vi "myRIOSpecPage_Template.vi"(10 "Spec Page Interface":T2, 11 "MetaDataObj in":refnum<class "MetaDataObj.lvclass">) -> (3 "MetaDataObj out":refnum<class "MetaDataObj.lvclass">)   [LabVIEW 2021, in "myRIOMetaDataObj.lvclass"]
uses:
  myRIOMetaDataObj.lvclass
  <resource>/dialog/NewProjectWizard/Icon Overlay/NI_NPW_Icon Overlay.lvlib
  <resource>/myRIO/Target Info.ctl
  WizardUIRef.ctl
  TargetListInfo.ctl
  TargetInfoHistory.ctl
  <vilib>/Utility/miscctls.llb/LVSelectionTypeDef.ctl
  AvailableTargets.ctl
  InternalErrorCodes.vi
  ModeFunctionality.ctl
  <vilib>/myRIO/Common/Instrument Driver Framework/Utilities/xctls/myRIO Device Button/myRIO Device Button.xctl
  <resource>/dialog/NewProjectWizard/MetaDataObj/MetaDataObj.lvclass
  <vilib>/Utility/cursorutil.llb/Set Cursor (Icon Pict).vi
  <vilib>/Platform/browser.llb/Open URL in Default Browser (string).vi
  p:/lvdist/win32/export/21.0/21.0.0f0/dist/resource/dialog/NewProjectWizard/MetaDataObj/MetaDataObj.lvclass
  p:/lvdist/win32/export/21.0/21.0.0f0/dist/ProjectTemplates/Source/myRIO/scripting/myRIOMetaDataObj/myRIOMetaDataObj.lvclass
  <resource>/dialog/NewProjectWizard/Spec Page Interface Confirm Quit.ctl
panel:
  in  "Project Name":string
  in  "Project Root":path
  in  "File Name Prefix (Optional)":string
  out "FPGA Personality Indicator":string
  out "myRIO Device Button":bool(xcontrol)
  in  "Personality Tags":u16(ring) items=["myRIO_FP_Default", "myRIO_FP_Throughput"]
  out "Mode Help Link":string
  out "FunctionalityArray":T1[](array[typedef])
  in  "FPGA Personality Selector":u16(ring) items=["Default", "High Throughput"]
  in  "Refresh Button":bool
  in  "Target Tab Control":enum32{"Target List Page", "IP Config Page"}(tab)
  in  "TargetList":i32(listbox) caption="Target List"
  in  "IP":string caption="IP Address or Hostname :"
  out "WarningMsg":string
  in  "AvailableTargets":T3
  # "Target"
  # "FPGA Personality"
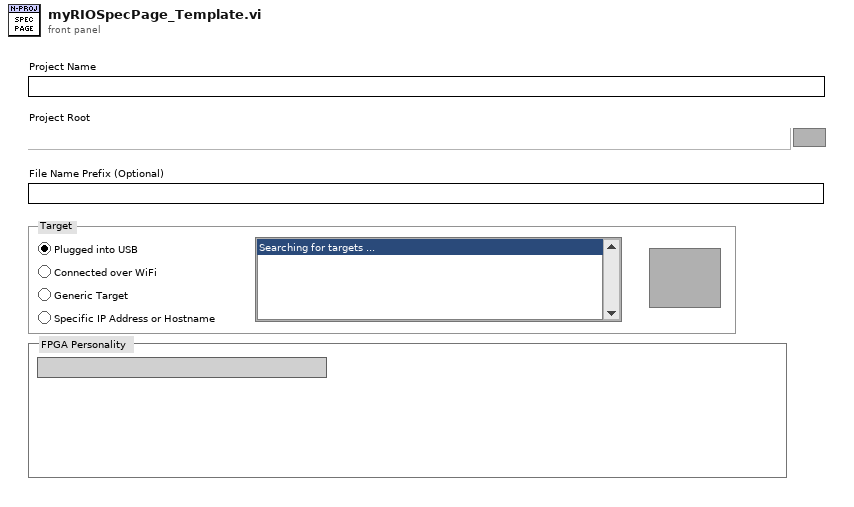
[diagram p1: front panel]
types:
  T1 = typedef "myRIOMetaDataObj.lvclass/ModeFunctionality.ctl" = cluster{"myRIOMode Functionality":u16, "SupportNumber":string}
  T2 = typedef "Spec Page Interface Confirm Quit.ctl" = cluster{"\"Tab Forward To\" Refnum":refnum<vi>, "\"Tab Backward To\" Refnum":refnum<vi>, "Errors":refnum<user-event>, "Quit":refnum<user-event>, "Additional Data":variant}
  T3 = typedef "myRIOMetaDataObj.lvclass/AvailableTargets.ctl" = enum32{"USBTarget", "WifiTarget", "NoSpecificTarget", "TargetIP"}
  T4 = typedef "myRIOMetaDataObj.lvclass/TargetInfoHistory.ctl" = cluster{"USBTargetList":T5, "WiFiTargetList":T5, "GenericTargetList":T5, "IPTargetList":cluster{"IP Error Out":errorcluster, "Target RT Info List":T6[]}}
  T5 = typedef "myRIOMetaDataObj.lvclass/TargetListInfo.ctl" = cluster{"TargetList":string[], "Value":i32, "Target RT Info List":T6[]}
  T6 = typedef "Target Info.ctl" = cluster{"MACAddr":string, "Hostname":string, "IPAddr":string, "SerialNum":string, "ProdID":u32}
  T7 = typedef "myRIOMetaDataObj.lvclass/WizardUIRef.ctl" = cluster{"Project Name":refnum<vi>, "Project Root":refnum<vi>, "File Name Prefix (Optional)":refnum<vi>, "AvailableTargets":refnum<vi>, "Target Tab Control":refnum<vi>, "TargetList":refnum<vi>, "IP":refnum<vi>, "Refresh":refnum<vi>, "FPGA Personality Selector":refnum<vi>, "FPGA Personality Indicator":refnum<vi>}
  T8 = cluster{"Quit":refnum<user-event>, "InitUI":refnum<user-event>, "ValidateUI":refnum<user-event>, "Show Overlay":refnum<user-event>, "Update Path":refnum<user-event>, "UpdateUI":refnum<user-event>}
  T9 = typedef "LVSelectionTypeDef.ctl" = cluster{"Selection Start":u32, "Selection End":u32}
  T10 = enum16{"Initial", "Get Channel Info Index by Name", "Get Channel Info by Index", "Get Channel Info by Img Index"}
  T11 = enum8{"Enabled", "Disabled", "Disabled and Grayed Out"}
  T12 = enum32{"USBTarget", "WifiTarget", "NoSpecificTarget", "TargetIP"}
  T13 = typedef "myRIOMetaDataObj.lvclass/IODetail.ctl" = cluster{"Channel Info Index":i8, "IO Number":i8}
  T14 = typedef "myRIOMetaDataObj.lvclass/ChannelInfo.ctl" = cluster{"Priority":u16, "Channel Shortcut":string, "Channel Description":string, "Channl Image Index":u16}
  T15 = typedef "LVPoint32TypeDef.ctl" = cluster{"Horizontal":i32, "Vertical":i32}
  T16 = typedef "lveventtype.ctl" = enum32{"Null", "Timeout", "Annotation Menu Selection", "Annotation Menu Selection?", "App Instance Close", "App Instance Close?", "Autoscale Range Change", "Bookmark Info Change", "Cell Edit", "Cell Edit?", "Cursor Grab", "Cursor Grab?", "Cursor Menu Selection", "Cursor Menu Selection?", "Cursor Move", "Cursor Release", "Data Change", "Direction Change", "Display State Change", "Drag Ended", "Drag Enter", "Drag Leave", "Drag Over", "Drag Source Update", "Drag Starting", "Drag Starting?", "Drop", "Exec State Change", "Key Down", "Key Down?", "Key Repeat", "Key Repeat?", "Key Up", "Listbox Double Click", "Menu Activation?", "Menu Selection (App)", "Menu Selection? (App)", "Menu Selection (User)", "Mouse Down", "Mouse Down?", "Mouse Enter", "Mouse Leave", "Mouse Move", "Mouse Up", "Mouse Wheel", "NI Security User Change (App)", "Pane Size", "Panel Close", "Panel Close?", "Panel Resize", "Plot Attribute Change", "Scale Range Change", "Shortcut Menu Activation?", "Shortcut Menu Selection (App)", "Shortcut Menu Selection? (App)", "Shortcut Menu Selection (User)", "Tree Double Click", "Tree Drag", "Tree Drag?", "Tree Drop", "Tree Drop?", "Tree Item Close", "Tree Item Close?", "Tree Item Open", "Tree Item Open?", "User Event", "Value Change"}
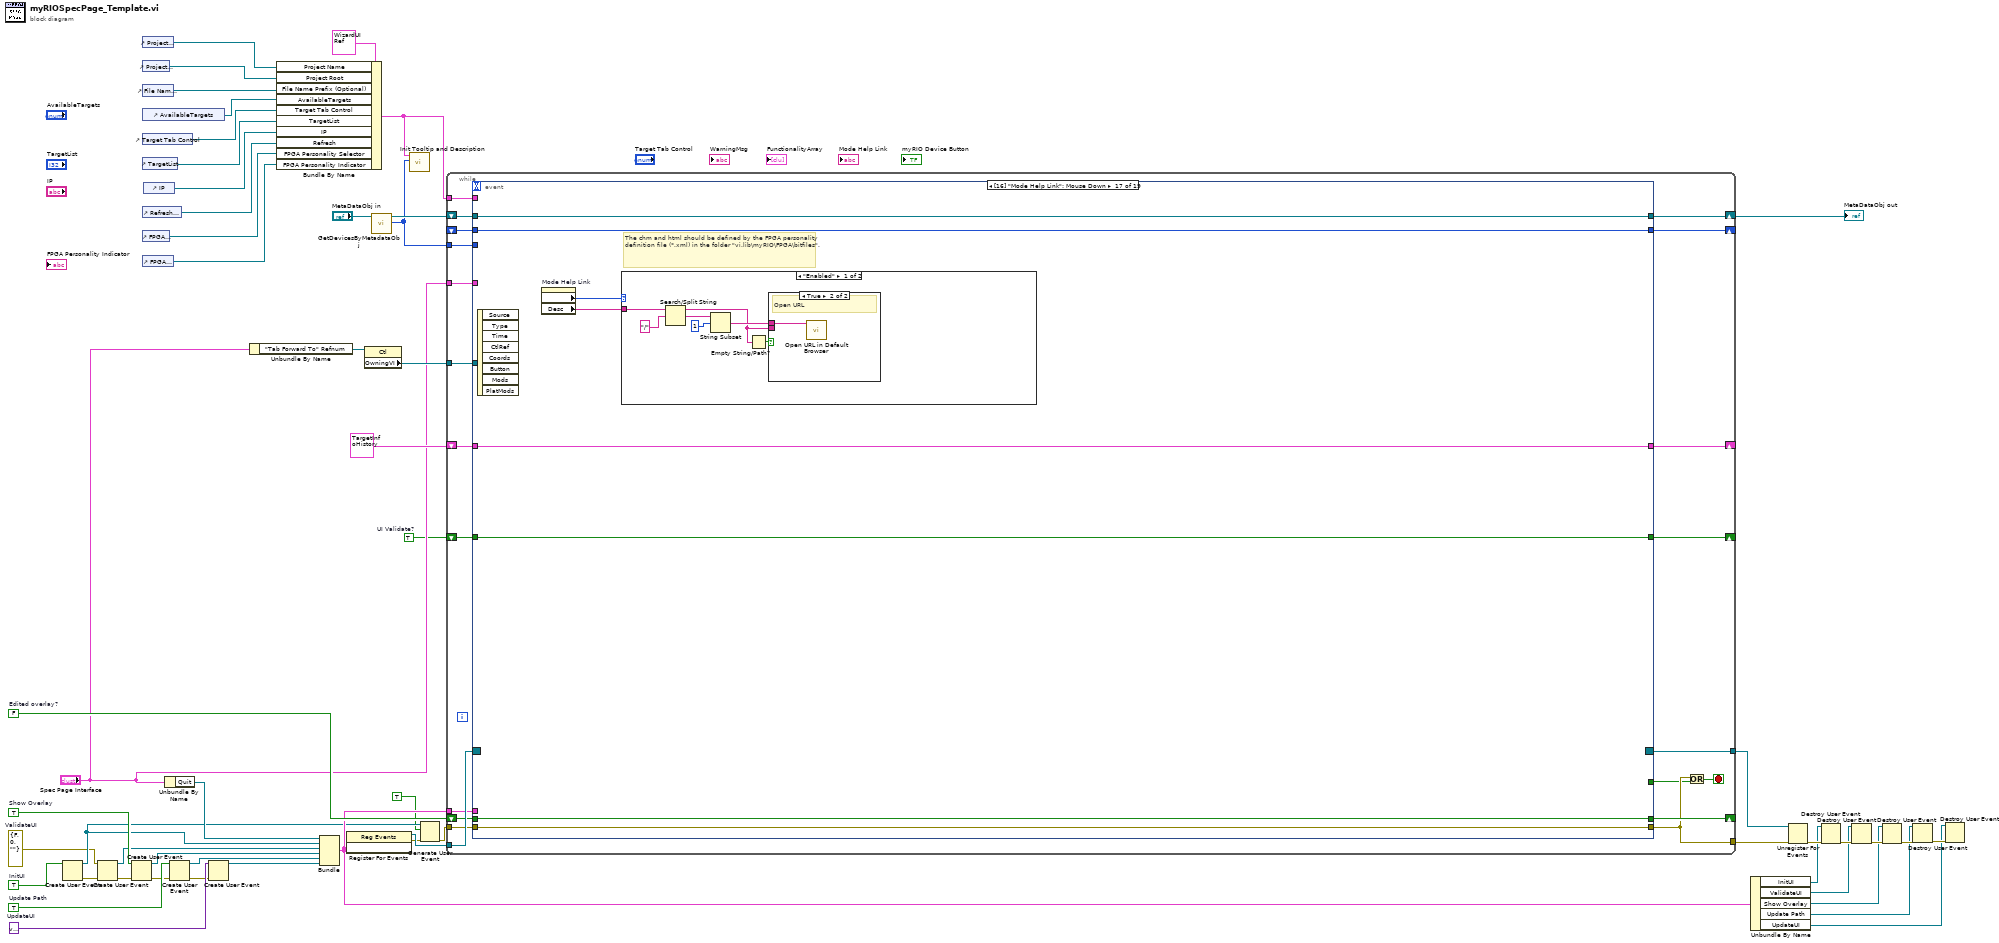
[diagram p0: block diagram]
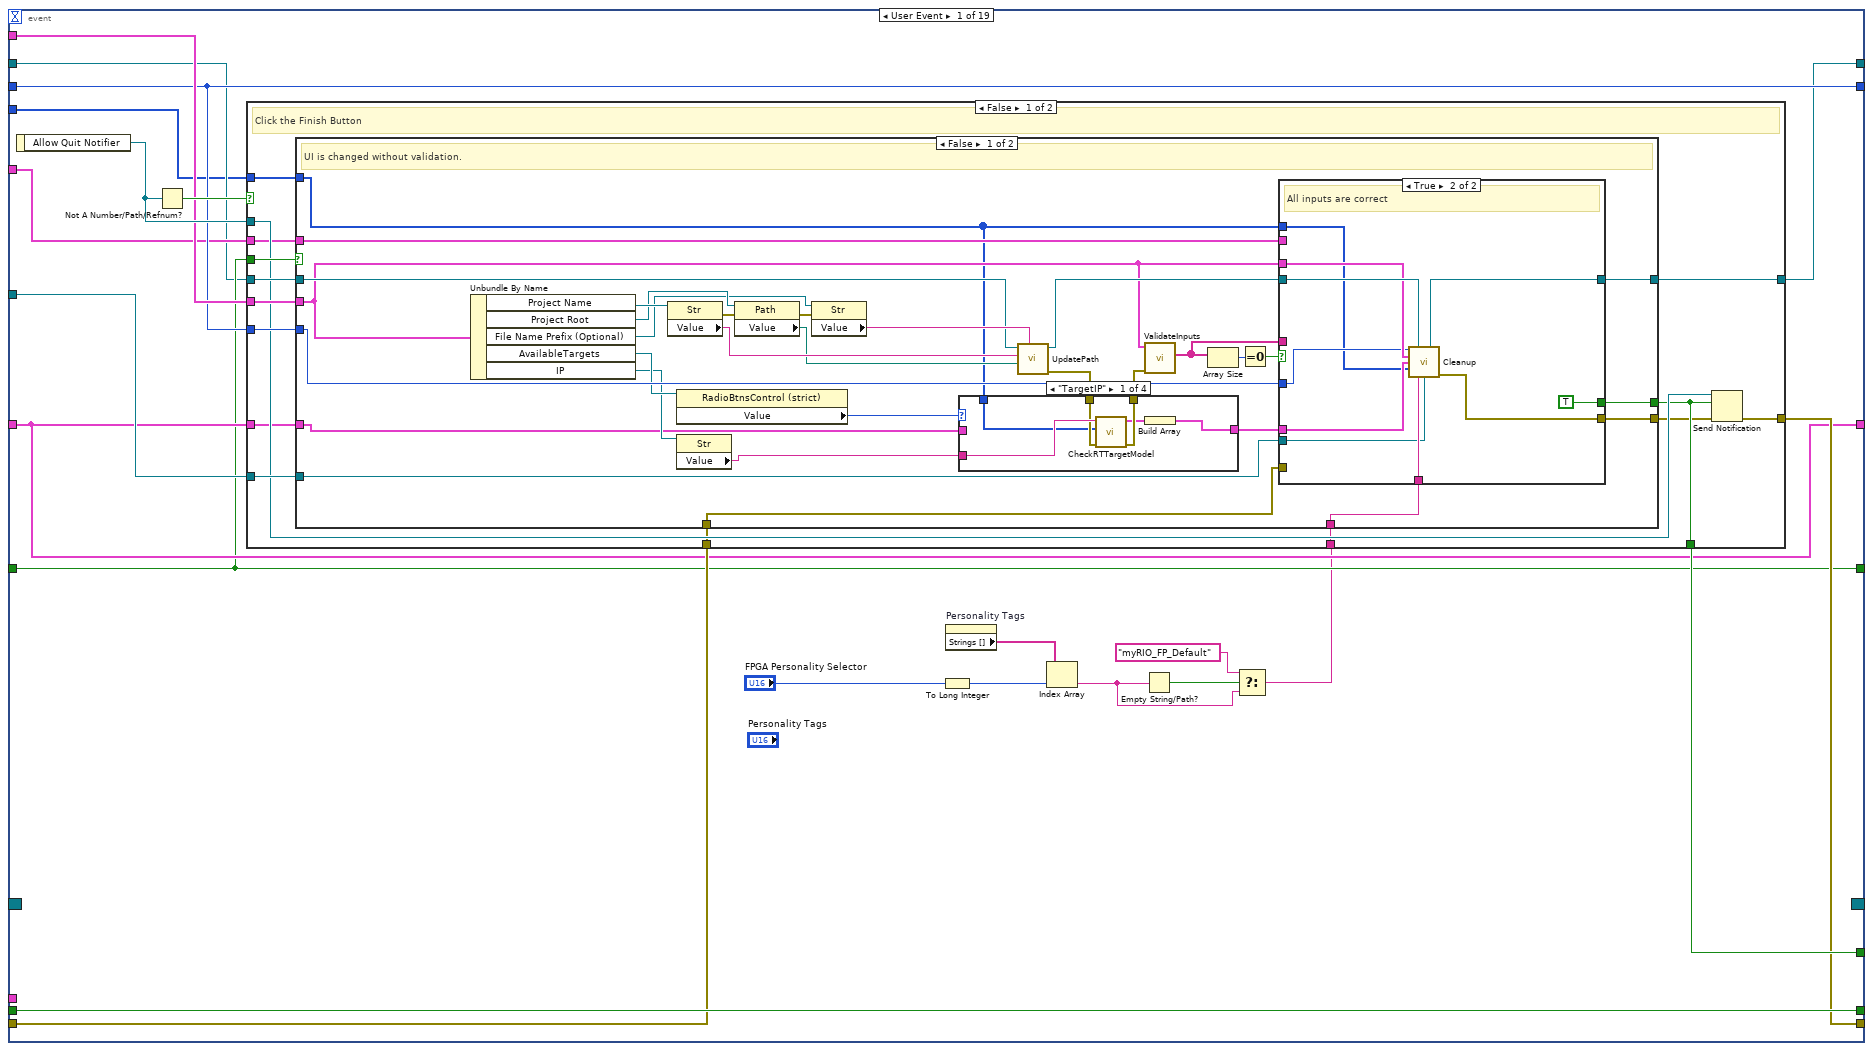
[diagram p2: hidden frame]
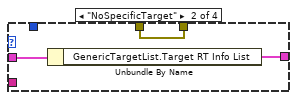
[diagram p3: hidden frame]
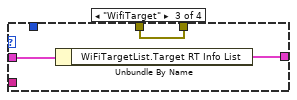
[diagram p4: hidden frame]
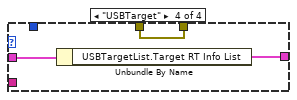
[diagram p5: hidden frame]
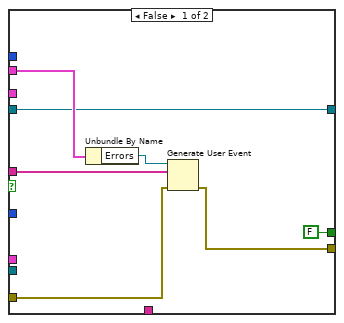
[diagram p6: hidden frame]
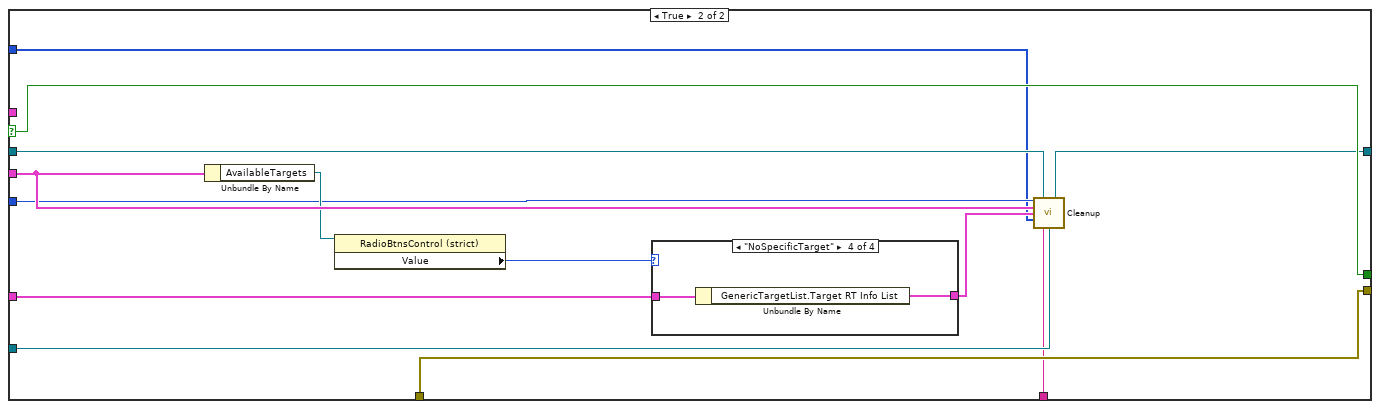
[diagram p7: hidden frame]
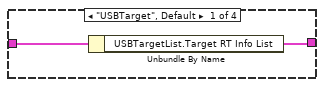
[diagram p8: hidden frame]
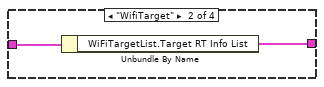
[diagram p9: hidden frame]
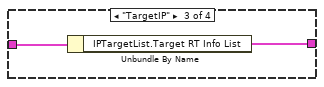
[diagram p10: hidden frame]
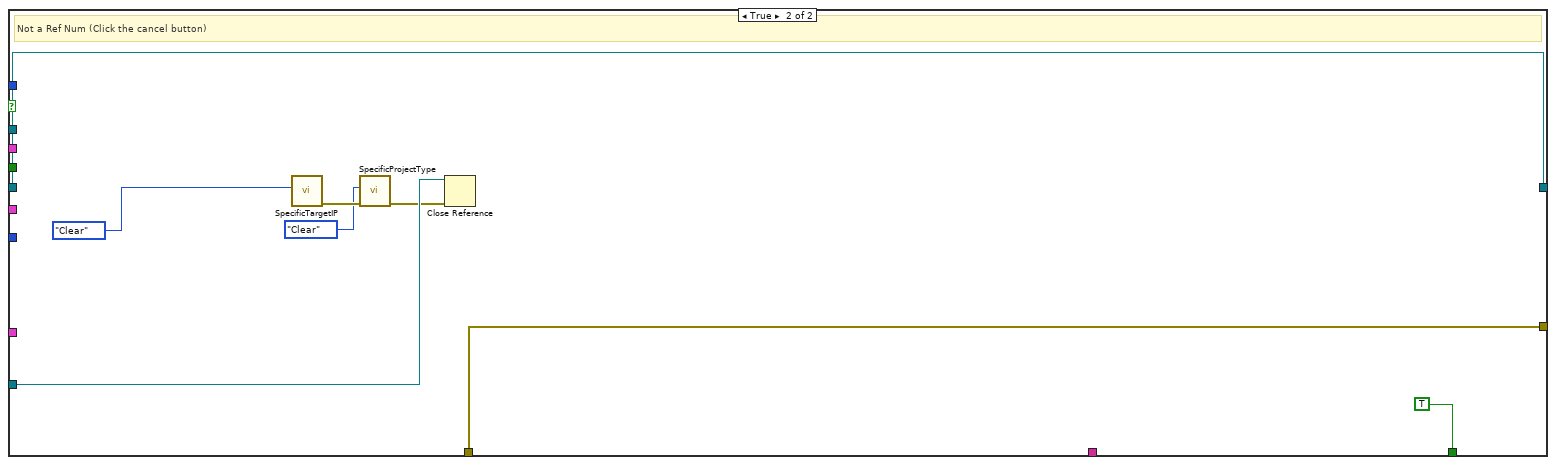
[diagram p11: hidden frame]
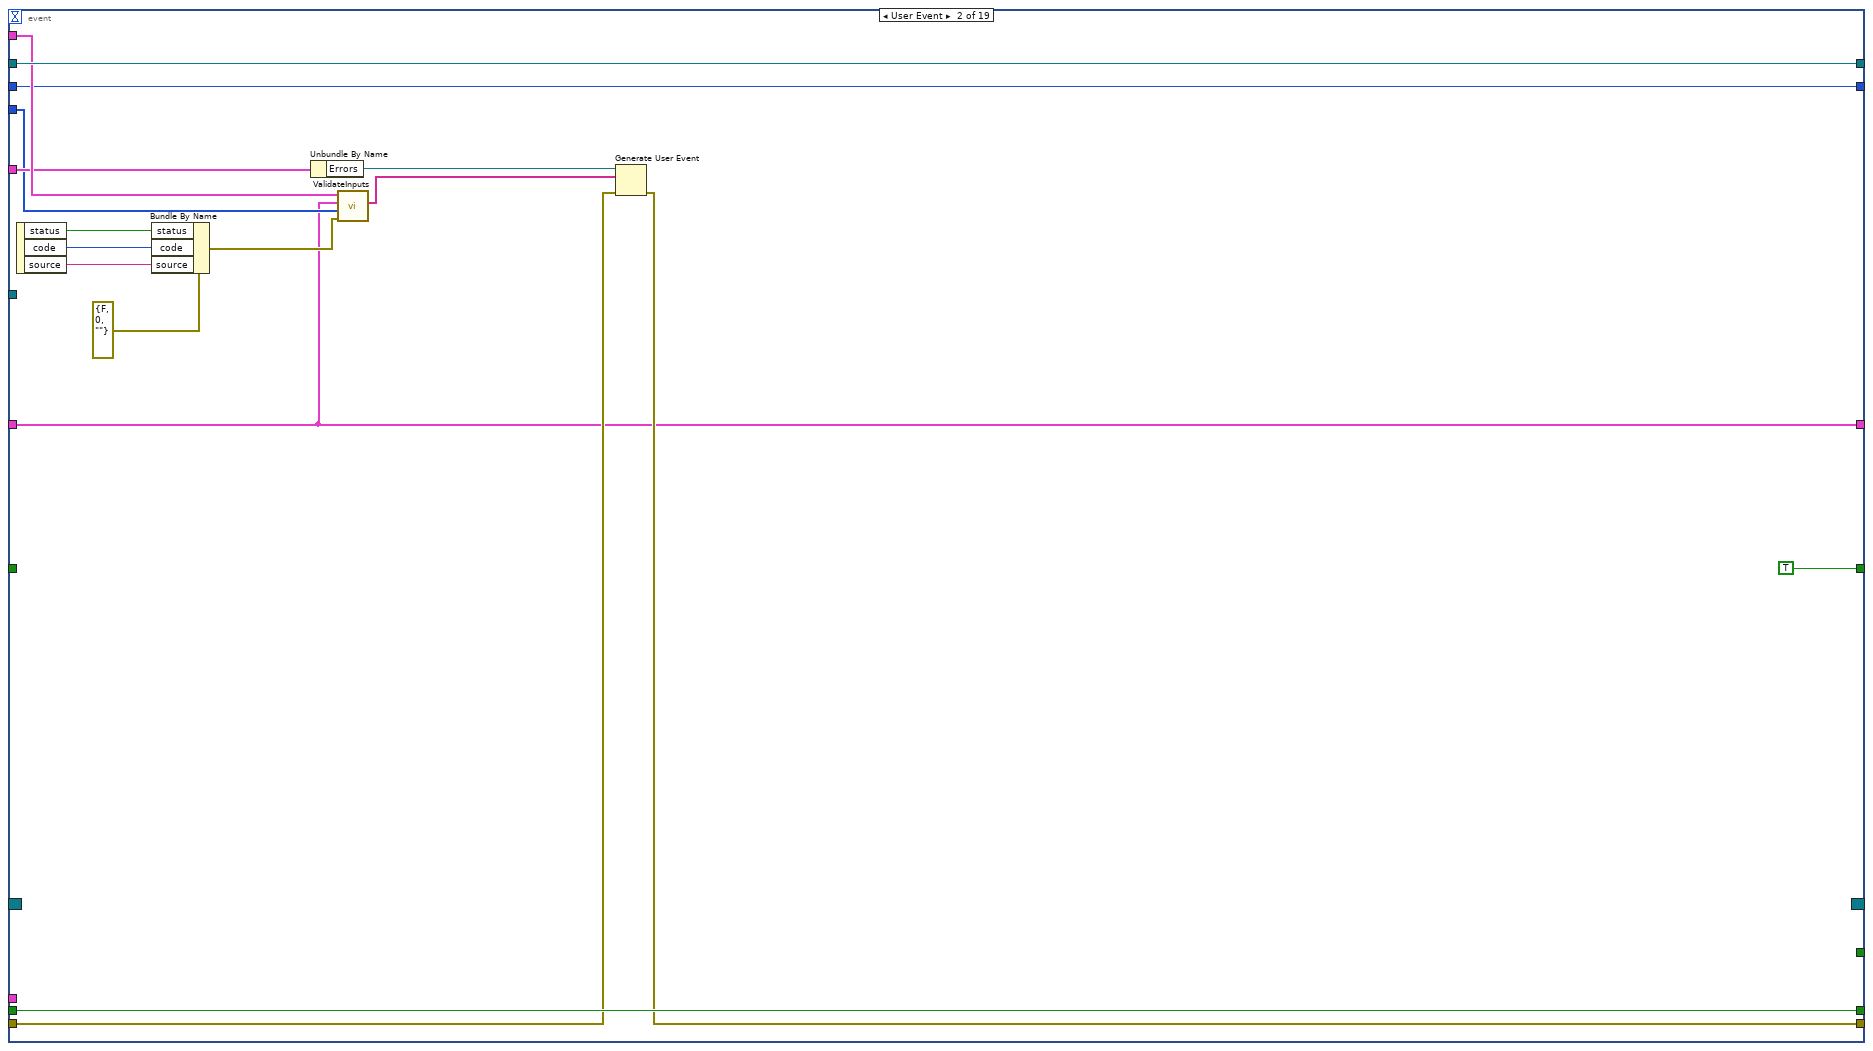
[diagram p12: hidden frame]
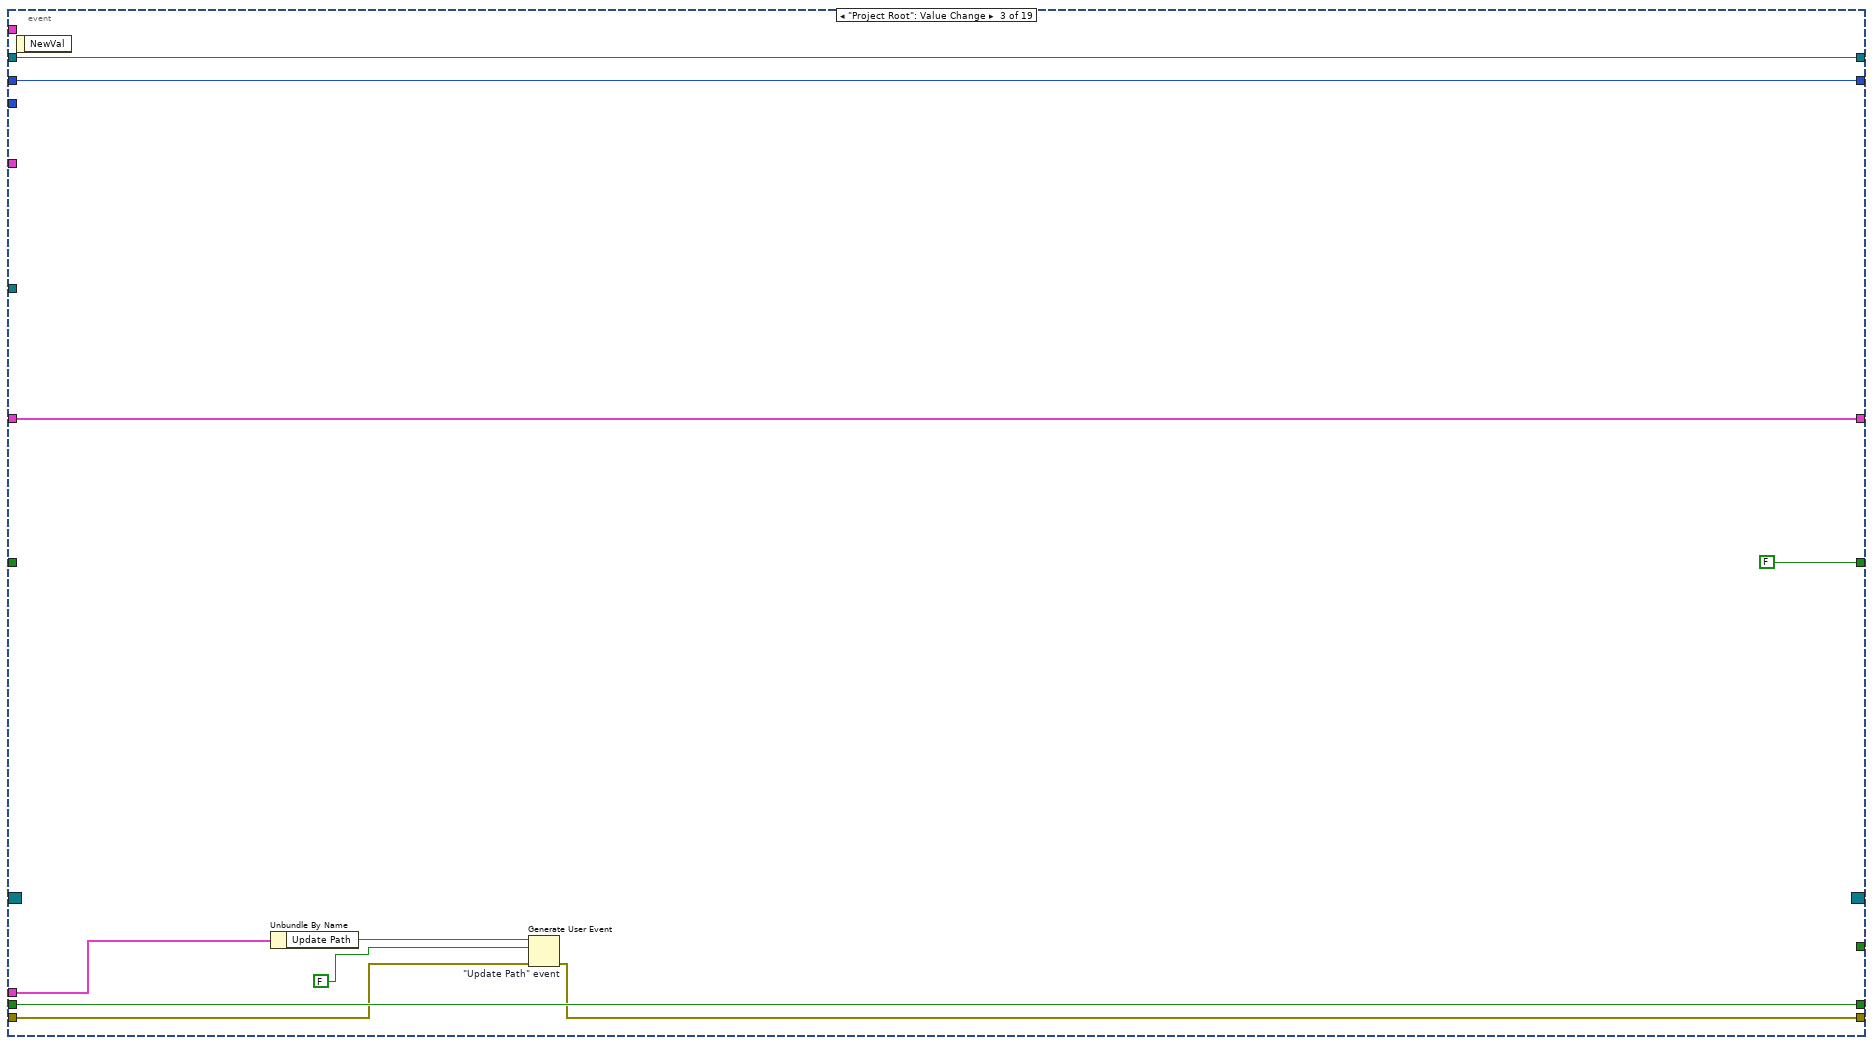
[diagram p13: hidden frame]
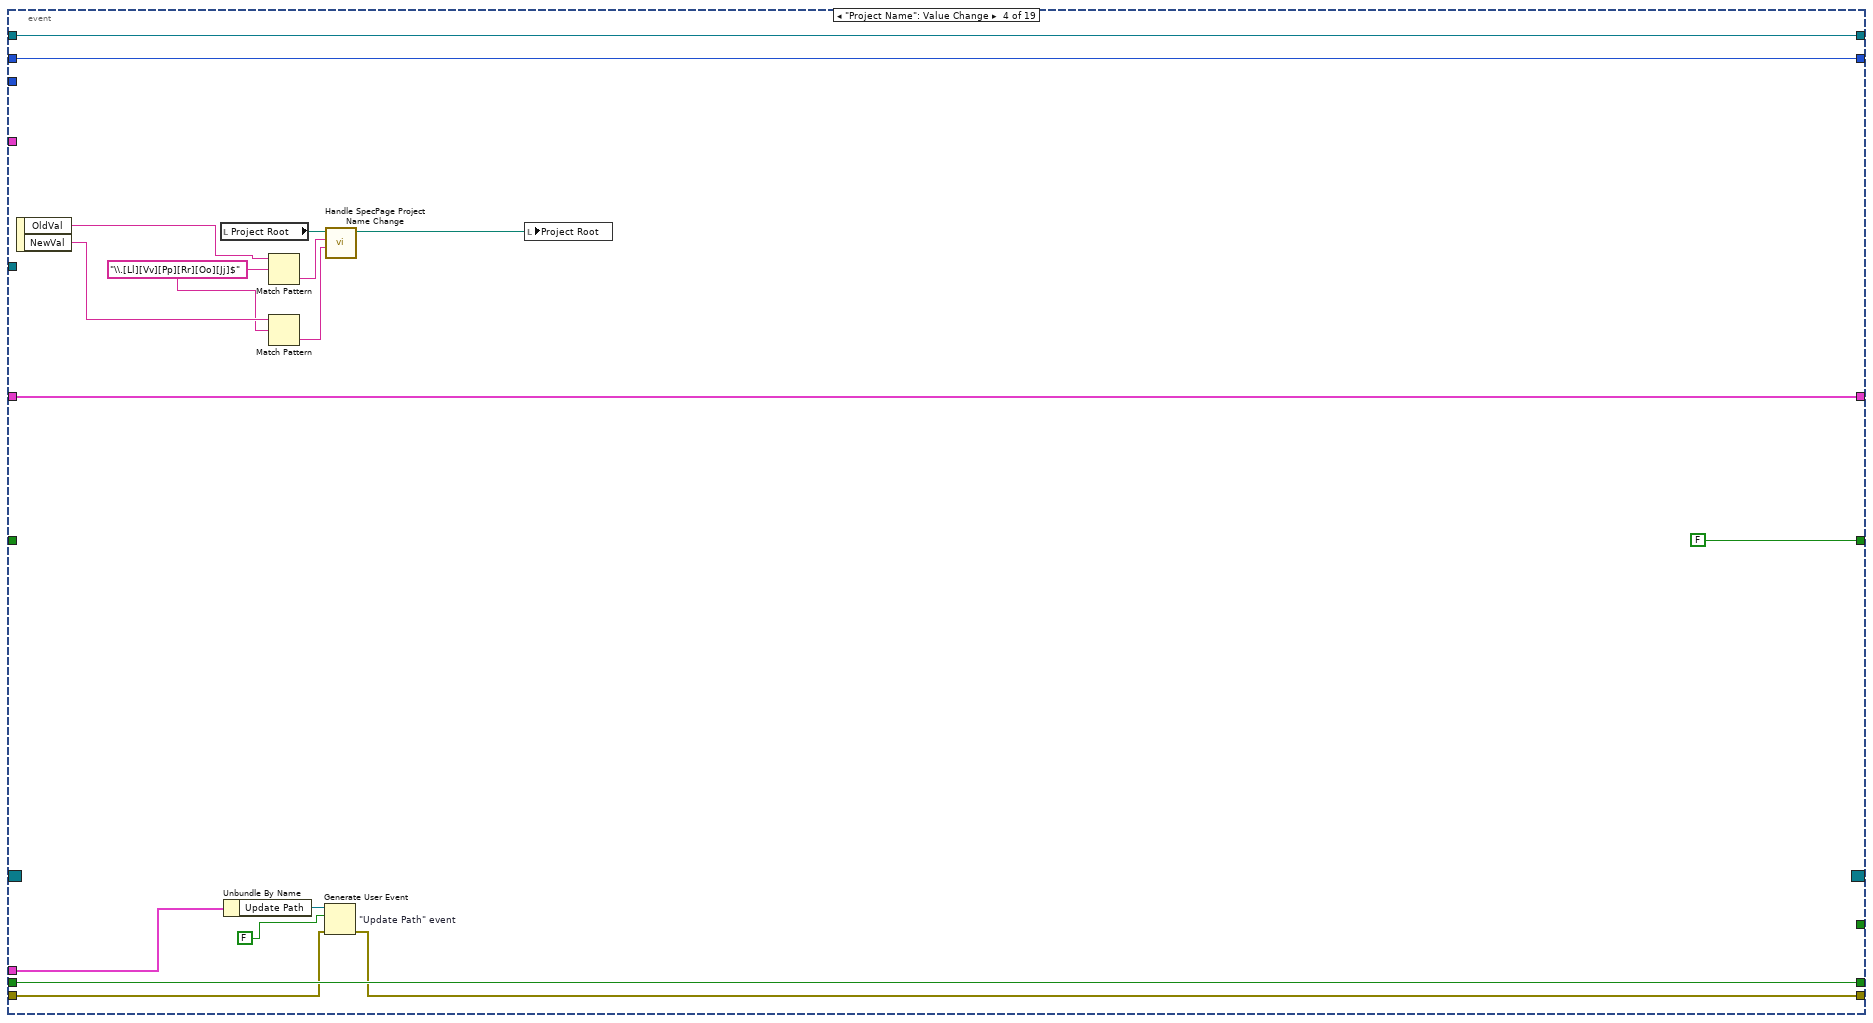
[diagram p14: hidden frame]
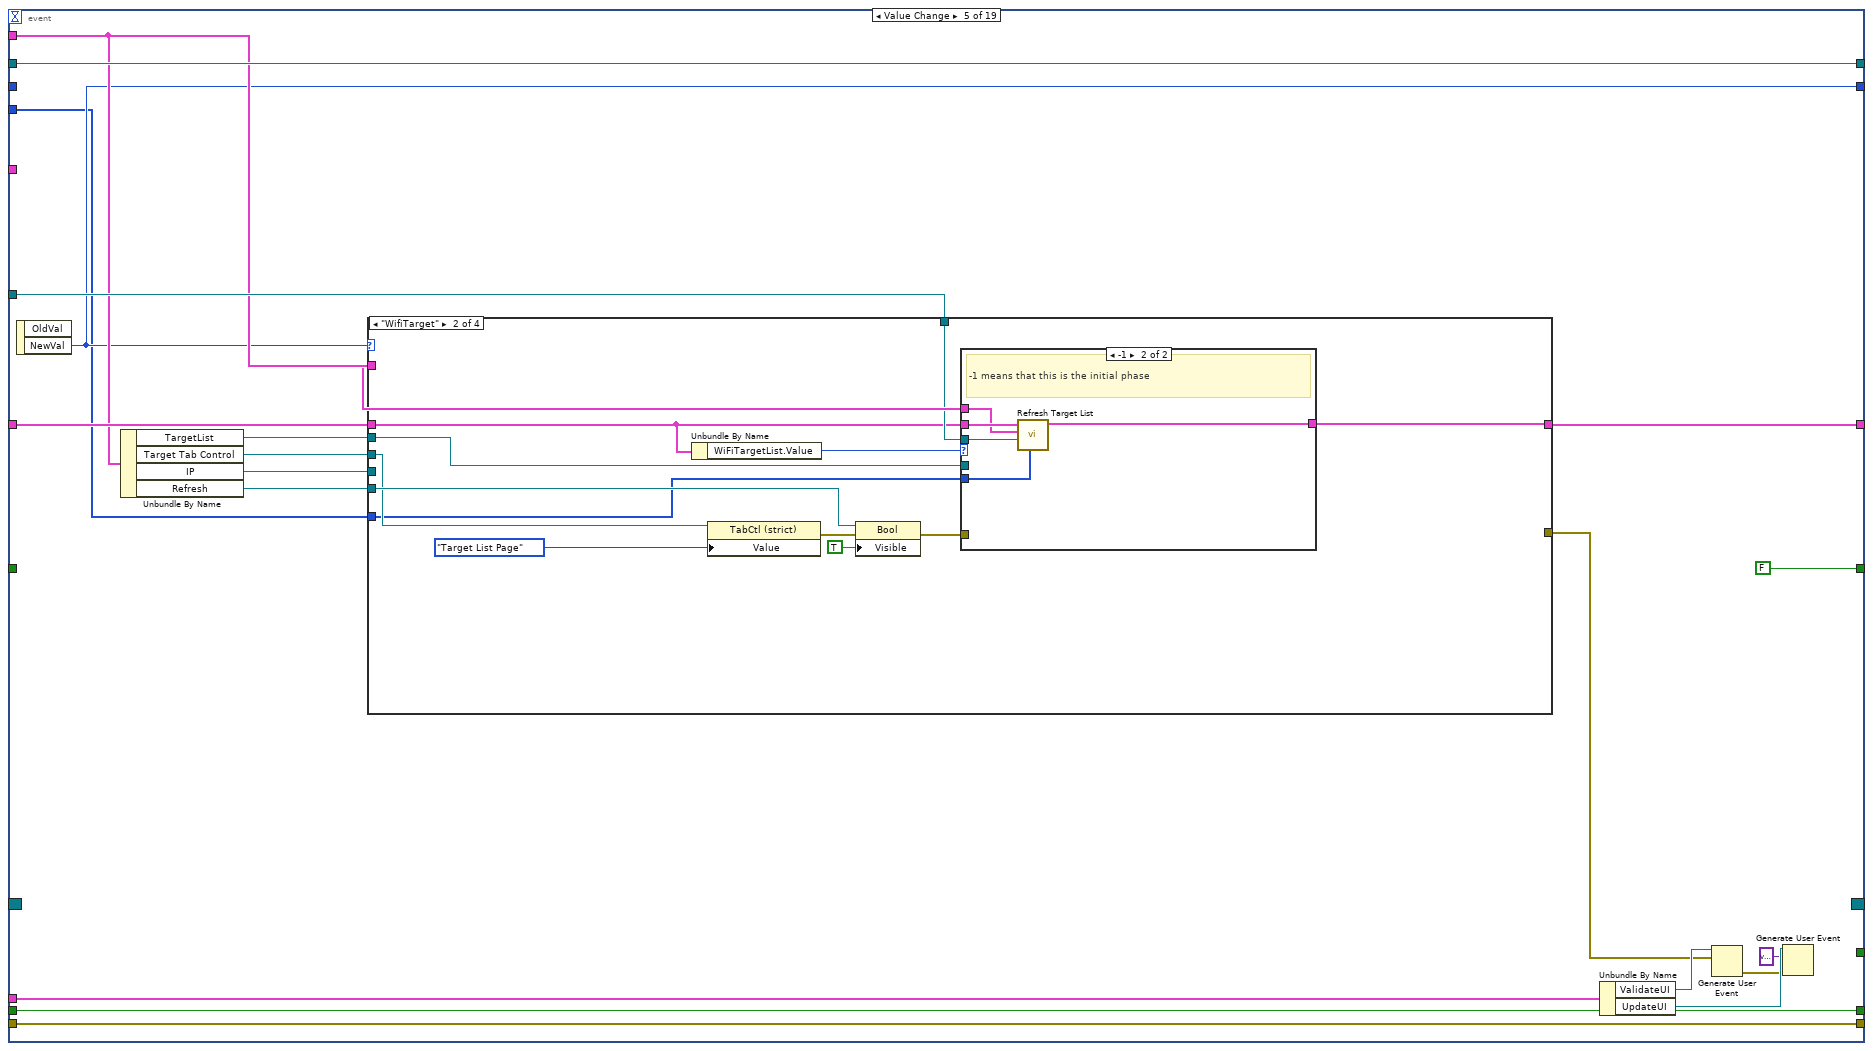
[diagram p15: hidden frame]
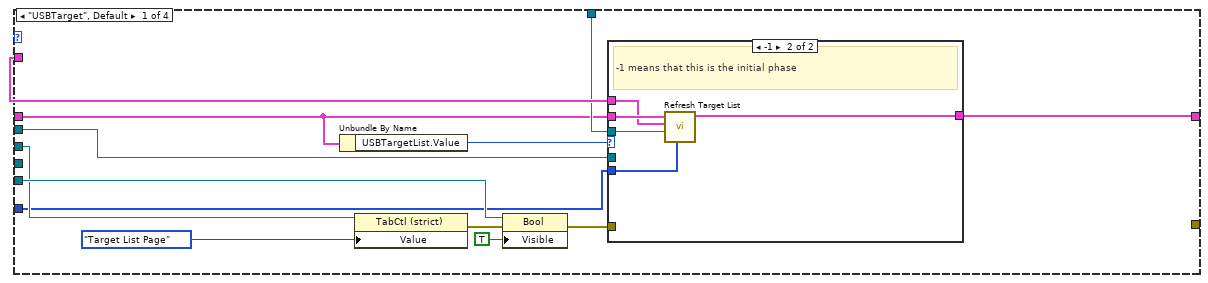
[diagram p16: hidden frame]
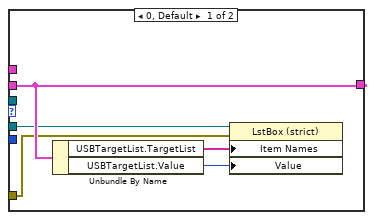
[diagram p17: hidden frame]
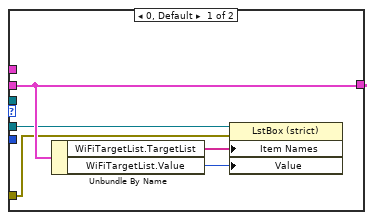
[diagram p18: hidden frame]
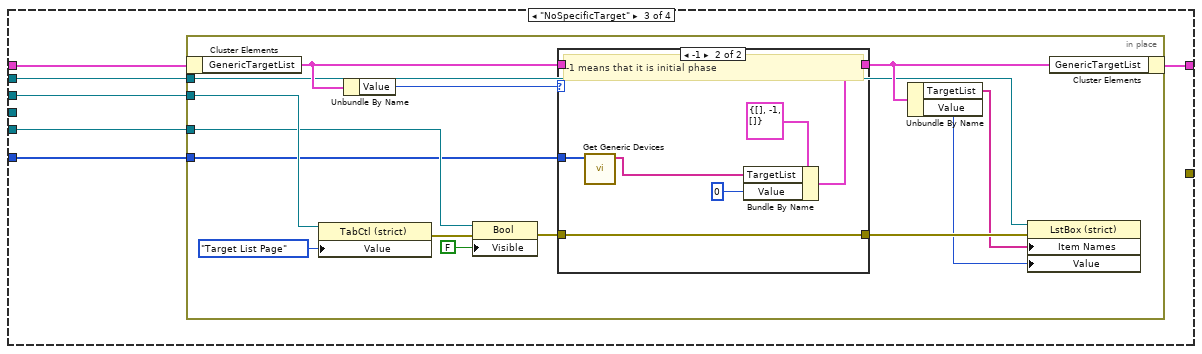
[diagram p19: hidden frame]
diagram:
  w12 = variant  # UpdateUI
  w15 = TRUE  # UI Validate?
  w14 = errorcluster {"status"=FALSE, "code"=0, "source"=""}  # ValidateUI
  w46 = TRUE  # InitUI
  w49 = FALSE  # Edited overlay?
  w48 = TRUE  # Show Overlay
  w53 = TRUE  # Update Path
  n1 = Create User Event(user event datatype=w46) -> (user event=w22:refnum<user-event>, error out=w45:errorcluster)  [unwired: 1 in]
  n2 = Create User Event(user event datatype=w14, error in=w45) -> (user event=w42:refnum<user-event>, error out=w44:errorcluster)
  n3 = Create User Event(user event datatype=w48, error in=w44) -> (user event=w41:refnum<user-event>, error out=w43:errorcluster)
  n4 = control-ref of="Project Name"() -> (w33:refnum<vi>)
  n5 = control-ref of="Project Root"() -> (w34:refnum<vi>)
  n6 = control-ref of="File Name Prefix (Optional)"() -> (w35:refnum<vi>)
  n7 = control-ref of="AvailableTargets"() -> (w7:refnum<vi>)
  n8 = control-ref of="Target Tab Control"() -> (w36:refnum<vi>)
  n9 = control-ref of="TargetList"() -> (w37:refnum<vi>)
  n10 = control-ref of="Refresh Button"() -> (w13:refnum<vi>)
  n11 = control-ref of="FPGA Personality Selector"() -> (w6:refnum<vi>)
  n12 = control-ref of="FPGA Personality Indicator"() -> (w5:refnum<vi>)
  n13 = control-ref of="IP"() -> (w38:refnum<vi>)
  n14 = Unbundle By Name("Spec Page Interface") -> ("Quit"=w39:refnum<user-event>)
  n15 = Create User Event(user event datatype=w53, error in=w43) -> (user event=w40:refnum<user-event>, error out=w11:errorcluster)
  n16 = Create User Event(user event datatype=w12, error in=w11) -> (user event=w10:refnum<user-event>)  [unwired: 1 out]
  n17 = Unbundle By Name("Spec Page Interface") -> ("\"Tab Forward To\" Refnum"=w20:refnum<vi>)
  n18 = Bundle By Name(cluster=T7 {"Project Name"=refnum, "Project Root"=refnum, "File Name Prefix (Optional)"=refnum, "AvailableTargets"=refnum, "Target Tab Control"=refnum, "TargetList"=refnum, "IP"=refnum, "Refresh"=refnum, "FPGA Personality Selector"=refnum, "FPGA Personality Indicator"=refnum} ("output cluster"), "Project Name"=w33, "Project Root"=w34, "File Name Prefix (Optional)"=w35, "AvailableTargets"=w7, "Target Tab Control"=w36, "TargetList"=w37, "IP"=w38, "Refresh"=w13, "FPGA Personality Selector"=w6, "FPGA Personality Indicator"=w5) -> (w4:T7)
  n19 = Bundle("Quit"=w39, "InitUI"=w22, "ValidateUI"=w42, "Show Overlay"=w41, "Update Path"=w40, "UpdateUI"=w10) -> (w31:T8)  [unwired: 1 in]
  n20 = register-events(w31) -> (reference out=w54:refnum<event-registration>, error out=w24:errorcluster)  [unwired: 2 in]
  n21 = property class="Ctl"(reference=w20) -> ("OwningVI"=w19:refnum<vi>)  [unwired: 1 in, 2 out]
  n22 = call "GetDevicesByMetadataObj.vi"("MetaDataObj in"="MetaDataObj in") -> ("Supported Devices"=w3:u32[], "MetaDataObj Out"=w8:refnum<class "MetaDataObj.lvclass">)  [unwired: 7 in, 2 out]
  n23 = call "Init Tooltip and Description.vi"("Supported Devices"=w3, "Main UI Ref Cluster"=w4) -> ()  [unwired: 10 in]
  n24 = Generate User Event(user event=w22, event data cluster=TRUE ("event data"), error in=w24) -> (error out=w23:errorcluster)  [unwired: 1 in, 1 out]
  n25 = while {
    tunnel: "Spec Page Interface" -> [w74]
    shift-right: [w73] -> w51
    shift-left: w8 -> [w72]
    tunnel: w54 -> [w75]
    shift-right: [w69] -> _
    shift-left: w49 -> [w70]
    shift-right: [w68] -> _
    shift-left: _ -> [w67]
    tunnel: w23 -> [w66]
    tunnel: w4 -> [w63]
    tunnel: [w65] -> w47
    tunnel: w31 -> [w64]
    tunnel: w19 -> [w62]
    tunnel: [w61] -> w18
    shift-right: [w59] -> _
    shift-left: T4 {"USBTargetList"={"TargetList"=[], "Value"=-1, "Target RT Info List"=[]}, "WiFiTargetList"={"TargetList"=[], "Value"=-1, "Target RT Info List"=[]}, "GenericTargetList"={"TargetList"=[], "Value"=-1, "Target RT Info List"=[]}, "IPTargetList"={"IP Error Out"={"status"=FALSE, "code"=0, "source"=""}, "Target RT Info List"=[]}} ("TargetInfoHistory") -> [w60]
    shift-right: [w58] -> _
    shift-left: w15 -> [w57]
    tunnel: w3 -> [w55]
    stop <- w71 stop-if-true
    n26 = event shown="[16] \"Mode Help Link\": Mouse Down" {
      selector: w75 -> [_ _ _ _ _ _ _ _ _ _ _ _ _ _ _ _ _ _ _]
      dyn-events: [_ _ _ _ _ _ _ _ _ _ _ _ _ _ _ _ _ _ _] -> w61
      timeout: _ -> [_ _ _ _ _ _ _ _ _ _ _ _ _ _ _ _ _ _ _]
      tunnel: w74 -> [w86 w216 _ _ _ _ _ _ _ _ w634 _ _ _ _ _ _ _ _]
      tunnel: [w89 w215 w224 w235 w266 w397 w485 w520 w582 w609 w635 w659 w664 w693 w762 w805 w813 w837 w875] -> w65
      tunnel: [w91 w221 w231 w244 w267 w383 w502 w536 w591 w602 w638 w662 w668 w695 w757 w804 w812 w836 w874] -> w73
      tunnel: w72 -> [w81 w221 w231 w244 w267 w410 w502 w536 w592 w603 w638 w662 w668 w695 w757 w804 w812 w836 w874]
      tunnel: w70 -> [w97 w220 w229 w245 w268 w427 w501 w537 w590 w614 w637 w661 w667 w694 w761 w803 w811 w835 w873]
      tunnel: [w97 w220 w229 w245 w268 w427 w501 w537 w590 w614 w637 w661 w667 w694 w761 w803 w811 w835 w873] -> w69
      tunnel: [w93 w214 w228 w238 w254 w396 w488 w526 w589 w613 w636 w650 w663 w687 w758 w802 w810 w834 w872] -> w68
      tunnel: w67 -> [w93 w214 w228 w238 _ _ w488 w526 w589 w613 w636 w650 w663 w687 w758 w802 w810 w834 w872]
      tunnel: w66 -> [w88 w213 w225 w234 w266 w380 w498 w533 w583 w610 w635 w660 w664 w693 w762 w805 w813 w837 w875]
      tunnel: w64 -> [_ _ w227 w237 w264 w405 w500 w535 w588 w612 _ w658 _ _ _ _ _ _ _]
      tunnel: w63 -> [w94 w217 _ _ w261 w393 w497 _ _ _ w633 w655 _ _ _ _ _ _ _]
      tunnel: w62 -> [w92 _ _ _ w265 w400 _ w532 _ _ _ w654 _ _ _ _ _ _ w868]
      tunnel: w60 -> [w87 w205 w223 w233 w263 w398 w493 w530 w581 w607 w632 w652 w666 w686 w759 w801 w808 w833 w871]
      tunnel: [w87 w205 w223 w233 w255 w398 w490 w527 w581 w607 w632 w651 w666 w686 w759 w801 w808 w833 w871] -> w59
      tunnel: [w82 TRUE FALSE ("UI Validate?") FALSE ("UI Validate?") FALSE FALSE ("UI Validate?") w494 FALSE ("UI Validate?") FALSE ("UI Validate?") w608 w631 FALSE ("UI Validate?") FALSE ("UI Validate?") w692 w760 w800 w809 w832 w870] -> w58
      tunnel: w57 -> [w82 _ _ _ _ _ _ _ _ w608 w631 _ _ w692 w760 w800 w809 w832 w870]
      tunnel: [w90 _ _ _ _ _ _ _ _ _ _ _ _ _ _ _ _ _ _] -> w56
      tunnel: w55 -> [w80 w206 _ _ w249 w377 _ w518 _ _ _ w649 _ w669 w751 _ _ _ _]
      event User Event {
        n27 = event-data() -> ("Allow Quit Notifier"=w95:refnum<notifier>)  [unwired: 1 in]
        n28 = Not A Number/Path/Refnum?(number/path/refnum=w95) -> (NaN/Path/Refnum?=w96:bool)
        n29 = To Long Integer(number="FPGA Personality Selector") -> (32bit integer=w83:i32)
        n30 = property on="Personality Tags" class="Ring (strict)"() -> ("Strings []"=w85:string[])  [unwired: 2 in, 2 out]
        n31 = Index Array(array=w85, index=w83) -> (element=w78:string)
        n32 = Empty String/Path?(string/path=w78) -> (empty?=w79:bool)
        n33 = Select(t="myRIO_FP_Default", s=w79, f=w78) -> (s? t:f=w76:string)
        n34 = case shown="False" w96 {
          tunnel: w82 -> [w112 _]
          tunnel: w95 -> [w107 _]
          tunnel: w94 -> [w111 _]
          tunnel: w93 -> [w110 _]
          tunnel: w92 -> [w109 w202]
          tunnel: w81 -> [w108 w204]
          tunnel: [w102 w204] -> w91
          tunnel: [w106 TRUE ("Quit")] -> w90
          tunnel: [w105 w197] -> w89
          tunnel: w88 -> [w103 w197]
          tunnel: w87 -> [w101 _]
          tunnel: w86 -> [w100 _]
          tunnel: w76 -> [w99 _]
          tunnel: w80 -> [w98 _]
          frame False {
            # "Click the Finish Button"
            n35 = case shown="False" w112 {
              selector: w112 -> [_ w187]
              tunnel: w111 -> [w124 w183]
              tunnel: w110 -> [w125 w178]
              tunnel: w109 -> [w123 w186]
              tunnel: w108 -> [w128 w185]
              tunnel: [w133 w187] -> w106
              tunnel: [w130 w188] -> w104
              tunnel: w103 -> [w129 w188]
              tunnel: [w127 w184] -> w102
              tunnel: w101 -> [w115 w180]
              tunnel: w100 -> [w131 _]
              tunnel: w99 -> [w114 w177]
              tunnel: w98 -> [w113 w176]
              frame False {
                # "UI is changed without validation."
                n36 = Unbundle By Name(w124) -> ("Project Name"=w143:refnum<vi>, "Project Root"=w142:refnum<vi>, "File Name Prefix (Optional)"=w139:refnum<vi>, "AvailableTargets"=w122:refnum<vi>, "IP"=w120:refnum<vi>)
                n37 = property class="Str"(reference=w143) -> (error out=w141:errorcluster, "Value"=w138:string)  [unwired: 1 in, 1 out]
                n38 = property class="RadioBtnsControl (strict)"(reference=w122) -> ("Value"=w121:T12)  [unwired: 1 in, 2 out]
                n39 = property class="Str"(reference=w120) -> ("Value"=w119:string)  [unwired: 1 in, 2 out]
                n40 = property class="Path"(reference=w142, error in=w141) -> (error out=w140:errorcluster, "Value"=w137:path)  [unwired: 1 out]
                n41 = property class="Str"(reference=w139, error in=w140) -> ("Value"=w136:string)  [unwired: 2 out]
                n42 = call "UpdatePath.vi"("File Name Prefix (Optional)"=w136, "Project Root"=w137, "Project Name"=w138, "MetaDataObj in"=w128) -> ("error out"=w118:errorcluster, "MetaDataObj out"=w126:refnum<class "MetaDataObj.lvclass">)  [unwired: 6 in]
                n43 = case shown="\"TargetIP\"" w121 {
                  tunnel: w119 -> [w149 _ _ _]
                  tunnel: w118 -> [w148 w150 w153 w156]
                  tunnel: [w147 w150 w153 w156] -> w117
                  tunnel: [w145 w151 w154 w157] -> w116
                  tunnel: w115 -> [_ w152 w155 w158]
                  tunnel: w113 -> [w144 _ _ _]
                  frame "TargetIP" {
                    n44 = call "CheckRTTargetModel.vi"("error in (no error)"=w148, "Supported Devices"=w144, "IP or Hostname"=w149) -> ("error out"=w147:errorcluster, "RT Target Info"=w146:T6)  [unwired: 7 in]
                    n45 = Build Array(w146) -> (w145:T6[])
                  }
                  frame "NoSpecificTarget" {
                    n46 = Unbundle By Name(w152) -> ("GenericTargetList.Target RT Info List"=w151:T6[])
                  }
                  frame "WifiTarget" {
                    n47 = Unbundle By Name(w155) -> ("WiFiTargetList.Target RT Info List"=w154:T6[])
                  }
                  frame "USBTarget" {
                    n48 = Unbundle By Name(w158) -> ("USBTargetList.Target RT Info List"=w157:T6[])
                  }
                }
                n49 = call "ValidateInputs.vi"("error in"=w117, "UI Ref Cluster"=w124) -> ("Error Message Array"=w132:string[])  [unwired: 7 in, 2 out]
                n50 = Array Size(array=w132) -> (size(s)=w135:i32)
                n51 = Equal To 0?(x=w135) -> (x = 0?=w134:bool)
                n52 = case shown="True" w134 {
                  tunnel: [FALSE TRUE] -> w133
                  tunnel: w132 -> [w165 _]
                  tunnel: w131 -> [w164 _]
                  tunnel: [w162 w174] -> w130
                  tunnel: w129 -> [w161 _]
                  tunnel: w126 -> [w159 w173]
                  tunnel: [w159 w172] -> w127
                  tunnel: w125 -> [_ w169]
                  tunnel: w124 -> [_ w171]
                  tunnel: w116 -> [_ w170]
                  tunnel: w123 -> [_ w166]
                  tunnel: w114 -> [_ w168]
                  tunnel: w113 -> [_ w167]
                  frame False {
                    n53 = Unbundle By Name(w164) -> ("Errors"=w163:refnum<user-event>)
                    n54 = Generate User Event(user event=w163, event data cluster=w165, error in=w161) -> (error out=w162:errorcluster)  [unwired: 1 in, 1 out]
                  }
                  frame True {
                    # "All inputs are correct"
                    n55 = call "Cleanup.vi"("Detected Type"=w169, "MetaDataObj in"=w173, "UI Ref Cluster"=w171, "Target Info"=w170, "Supported Devices"=w167, "Target FPGA Personality"=w168, "Owning VI Ref"=w166) -> ("MetaDataObj out"=w172:refnum<class "MetaDataObj.lvclass">, "error out"=w174:errorcluster)  [unwired: 7 in]
                  }
                }
              }
              frame True {
                n56 = Unbundle By Name(w183) -> ("AvailableTargets"=w182:refnum<vi>)
                n57 = property class="RadioBtnsControl (strict)"(reference=w182) -> ("Value"=w181:T12)  [unwired: 1 in, 2 out]
                n58 = case shown="\"NoSpecificTarget\"" w181 {
                  tunnel: w180 -> [w190 w192 w194 w196]
                  tunnel: [w189 w191 w193 w195] -> w179
                  frame "USBTarget", Default {
                    n59 = Unbundle By Name(w190) -> ("USBTargetList.Target RT Info List"=w189:T6[])
                  }
                  frame "WifiTarget" {
                    n60 = Unbundle By Name(w192) -> ("WiFiTargetList.Target RT Info List"=w191:T6[])
                  }
                  frame "TargetIP" {
                    n61 = Unbundle By Name(w194) -> ("IPTargetList.Target RT Info List"=w193:T6[])
                  }
                  frame "NoSpecificTarget" {
                    n62 = Unbundle By Name(w196) -> ("GenericTargetList.Target RT Info List"=w195:T6[])
                  }
                }
                n63 = call "Cleanup.vi"("Detected Type"=w178, "MetaDataObj in"=w185, "UI Ref Cluster"=w183, "Target Info"=w179, "Supported Devices"=w176, "Target FPGA Personality"=w177, "Owning VI Ref"=w186) -> ("MetaDataObj out"=w184:refnum<class "MetaDataObj.lvclass">)  [unwired: 7 in, 1 out]
              }
            }
            n64 = Send Notification(notification=w106, notifier=w107, error in (no error)=w104) -> (error out=w105:errorcluster)  [unwired: 1 out]
          }
          frame True {
            # "Not a Ref Num (Click the cancel button)"
            n65 = call "SpecificTargetIP.vi"("Action"=enum16{"Clear", "Get", "Set"}."Clear") -> ("error out"=w201:errorcluster)  [unwired: 9 in, 1 out]
            n66 = call "SpecificProjectType.vi"("error in (no error)"=w201, "Action"=enum16{"Clear", "Get", "Set"}."Clear") -> ("error out"=w200:errorcluster)  [unwired: 6 in, 3 out]
            n67 = Close Reference(reference=w202, error in (no error)=w200) -> ()  [unwired: 1 out]
          }
        }
      }
      event User Event {
        n68 = event-data() -> ("status"=w210:bool, "code"=w209:i32, "source"=w208:string)  [unwired: 1 in]
        n69 = Bundle By Name(cluster=errorcluster {"status"=FALSE, "code"=0, "source"=""} ("error out"), "status"=w210, "code"=w209, "source"=w208) -> (w207:errorcluster)
        n70 = Unbundle By Name(w216) -> ("Errors"=w219:refnum<user-event>)
        n71 = call "ValidateInputs.vi"("error in"=w207, "Supported Devices"=w206, "TargetInfoHistory"=w205, "UI Ref Cluster"=w217) -> ("Error Message Array"=w218:string[])  [unwired: 5 in, 2 out]
        n72 = Generate User Event(user event=w219, event data cluster=w218, error in=w213) -> (error out=w215:errorcluster)  [unwired: 1 in, 1 out]
      }
      event "Project Root": Value Change {
        n73 = event-data() -> ()  [unwired: 1 in, 1 out]
        n74 = Unbundle By Name(w227) -> ("Update Path"=w226:refnum<user-event>)
        n75 = Generate User Event "\"Update Path\" event"(user event=w226, event data cluster=FALSE ("event data"), error in=w225) -> (error out=w224:errorcluster)  [unwired: 1 in, 1 out]
      }
      event "Project Name": Value Change {
        w239 = "\\.[Ll][Vv][Pp][Rr][Oo][Jj]$" ("regular expression")
        n76 = event-data() -> ("OldVal"=w241:string, "NewVal"=w243:string)  [unwired: 1 in]
        n77 = local read "Project Root"() -> (w248:path)
        n78 = Unbundle By Name(w237) -> ("Update Path"=w236:refnum<user-event>)
        n79 = Match Pattern(string=w241, regular expression=w239) -> (before substring=w240:string)  [unwired: 1 in, 3 out]
        n80 = Match Pattern(string=w243, regular expression=w239) -> (before substring=w242:string)  [unwired: 1 in, 3 out]
        n81 = Generate User Event "\"Update Path\" event"(user event=w236, event data cluster=FALSE ("event data"), error in=w234) -> (error out=w235:errorcluster)  [unwired: 1 in, 1 out]
        n82 = call <resource>:"Handle SpecPage Project Name Change.vi"("Project Name New Value"=w242, "Project Name Old Value"=w240, "Project Root in"=w248) -> ("Project Root out"=w247:path)  [unwired: 8 in]
        n83 = local write "Project Root"(w247) -> ()
      }
      event Value Change {
        n84 = event-data() -> ("NewVal"=w254:T3)  [unwired: 1 in, 1 out]
        n85 = Unbundle By Name(w261) -> ("TargetList"=w257:refnum<vi>, "Target Tab Control"=w260:refnum<vi>, "IP"=w259:refnum<vi>, "Refresh"=w258:refnum<vi>)
        n86 = case shown="\"WifiTarget\"" w254 {
          tunnel: w261 -> [w278 w301 _ _]
          tunnel: w263 -> [w276 w298 w320 w352]
          tunnel: [w270 w299 w319 w352] -> w255
          tunnel: w265 -> [w277 w300 _ _]
          tunnel: [_ _ _ w360] -> w253
          tunnel: w260 -> [w273 w295 w318 w354]
          tunnel: w259 -> [_ _ _ w353]
          tunnel: w258 -> [w274 w296 w316 w351]
          tunnel: w257 -> [w272 w294 w317 _]
          tunnel: w249 -> [w269 w292 w315 _]
          frame "USBTarget", Default {
            n87 = Unbundle By Name(w276) -> ("USBTargetList.Value"=w275:i32)
            n88 = property class="TabCtl (strict)"(reference=w273, "Value"=enum32{"Target List Page", "IP Config Page"}."Target List Page") -> (error out=w279:errorcluster)  [unwired: 1 in, 1 out]
            n89 = property class="Bool"(reference=w274, error in=w279, "Visible"=TRUE) -> (error out=w271:errorcluster)  [unwired: 1 out]
            n90 = case shown="-1" w275 {
              tunnel: w276 -> [w284 w291]
              tunnel: [w284 w288] -> w270
              tunnel: w278 -> [_ w290]
              tunnel: w277 -> [_ w289]
              tunnel: w272 -> [w283 _]
              tunnel: w271 -> [w282 _]
              tunnel: w269 -> [_ w287]
              frame 0, Default {
                n91 = Unbundle By Name(w284) -> ("USBTargetList.TargetList"=w285:string[], "USBTargetList.Value"=w286:i32)
                n92 = property class="LstBox (strict)"(reference=w283, error in=w282, "Item Names"=w285, "Value"=w286) -> ()  [unwired: 2 out]
              }
              frame -1 {
                # "-1 means that this is the initial phase"
                n93 = call "Refresh Target List.vi"("Supported Devices"=w287, "OwningVI Ref"=w289, "UI Ref Cluster"=w290, "Target Info Cache"=w291) -> ("Target Info Cache Output"=w288:T4)  [unwired: 6 in, 1 out]
              }
            }
          }
          frame "WifiTarget" {
            n94 = Unbundle By Name(w298) -> ("WiFiTargetList.Value"=w297:i32)
            n95 = property class="TabCtl (strict)"(reference=w295, "Value"=enum32{"Target List Page", "IP Config Page"}."Target List Page") -> (error out=w302:errorcluster)  [unwired: 1 in, 1 out]
            n96 = property class="Bool"(reference=w296, error in=w302, "Visible"=TRUE) -> (error out=w293:errorcluster)  [unwired: 1 out]
            n97 = case shown="-1" w297 {
              tunnel: w298 -> [w307 w314]
              tunnel: [w307 w311] -> w299
              tunnel: w301 -> [_ w313]
              tunnel: w300 -> [_ w312]
              tunnel: w294 -> [w306 _]
              tunnel: w293 -> [w305 _]
              tunnel: w292 -> [_ w310]
              frame 0, Default {
                n98 = Unbundle By Name(w307) -> ("WiFiTargetList.TargetList"=w308:string[], "WiFiTargetList.Value"=w309:i32)
                n99 = property class="LstBox (strict)"(reference=w306, error in=w305, "Item Names"=w308, "Value"=w309) -> ()  [unwired: 2 out]
              }
              frame -1 {
                # "-1 means that this is the initial phase"
                n100 = call "Refresh Target List.vi"("Supported Devices"=w310, "OwningVI Ref"=w312, "UI Ref Cluster"=w313, "Target Info Cache"=w314) -> ("Target Info Cache Output"=w311:T4)  [unwired: 6 in, 1 out]
              }
            }
          }
          frame "NoSpecificTarget" {
            n101 = in-place {
              in-place-border: w318 -> [w324]
              in-place-border: w317 -> [w323]
              in-place-border: w316 -> [w322]
              in-place-border: w315 -> [w321]
              n102 = in-place-cluster #1(w320) -> ("GenericTargetList"=w329:T5)
              n103 = property class="TabCtl (strict)"(reference=w324, "Value"=enum32{"Target List Page", "IP Config Page"}."Target List Page") -> (error out=w332:errorcluster)  [unwired: 1 in, 1 out]
              n104 = Unbundle By Name(w329) -> ("Value"=w333:i32)
              n105 = property class="Bool"(reference=w322, error in=w332, "Visible"=FALSE) -> (error out=w330:errorcluster)  [unwired: 1 out]
              n106 = case shown="-1" w333 {
                tunnel: w329 -> [w336 _]
                tunnel: [w336 w341] -> w328
                tunnel: w330 -> [w335 w339]
                tunnel: [w335 w339] -> w327
                tunnel: w321 -> [_ w338]
                frame 0, Default {
                }
                frame -1 {
                  # "-1 means that it is initial phase"
                  n107 = call "Get Generic Devices.vi"("Supported Device Code"=w338) -> ("Supported Device Full Name"=w337:string[])  [unwired: 10 in]
                  n108 = Bundle By Name(cluster=T5 {"TargetList"=[], "Value"=-1, "Target RT Info List"=[]} ("TargetListInfo"), "TargetList"=w337, "Value"=0) -> (w341:T5)
                }
              }
              n109 = Unbundle By Name(w328) -> ("TargetList"=w326:string[], "Value"=w325:i32)
              n110 = property class="LstBox (strict)"(reference=w323, error in=w327, "Item Names"=w326, "Value"=w325) -> ()  [unwired: 2 out]
              n111 = in-place-cluster #1("GenericTargetList"=w328) -> (w319:T4)
            }
          }
          frame "TargetIP" {
            n112 = property class="Bool"(reference=w351, "Visible"=FALSE) -> (error out=w349:errorcluster)  [unwired: 1 in, 1 out]
            n113 = Unbundle By Name(w352) -> ("IPTargetList.IP Error Out"=w360:errorcluster)
            n114 = property class="TabCtl (strict)"(reference=w354, error in=w349, "Value"=enum32{"Target List Page", "IP Config Page"}."IP Config Page") -> (error out=w359:errorcluster)  [unwired: 1 out]
            n115 = property class="Str"(reference=w353, error in=w359, "Key Focus"=TRUE) -> (reference out=w357:refnum<vi>, error out=w356:errorcluster, "Value"=w348:string)
            n116 = Empty String/Path?(string/path=w348) -> (empty?=w355:bool)
            n117 = case shown="False" w355 {
              tunnel: w357 -> [w363 w371]
              tunnel: w356 -> [w362 w370]
              tunnel: [w364 w368] -> w346
              tunnel: w348 -> [w365 _]
              tunnel: [w362 w367] -> w344
              tunnel: [w363 w366] -> w343
              frame False {
                n118 = String Length(string=w365) -> (length=w364:i32)
              }
              frame True {
                w369 = "0.0.0.0" ("Value")
                # "The IP Address is empty"
                n119 = String Length(string=w369) -> (length=w368:i32)
                n120 = property class="Str"(reference=w371, error in=w370, "Val(Sgnl)"=w369) -> (reference out=w366:refnum<vi>, error out=w367:errorcluster)
              }
            }
            n121 = Bundle By Name(cluster=T9 {"Selection Start"=0, "Selection End"=0} ("Text.Selection"), "Selection End"=w346) -> (w345:T9)
            n122 = property class="Str"(reference=w343, error in=w344, "Text.Selection"=w345) -> ()  [unwired: 2 out]
          }
        }
        n123 = Unbundle By Name(w264) -> ("ValidateUI"=w262:refnum<user-event>, "UpdateUI"=w252:refnum<user-event>)
        n124 = Generate User Event(user event=w262, event data cluster=w253) -> (error out=w250:errorcluster)  [unwired: 2 in, 1 out]
        n125 = Generate User Event(user event=w252, event data cluster=variant ("event data"), error in=w250) -> ()  [unwired: 1 in, 2 out]
      }
      event User Event {
        w389 = refnum<vi> refnum  # Boolean
        w417 = ""
        w424 = TRUE
        # "Initilize device button to empty"
        n126 = event-data() -> ()  [unwired: 1 in, 1 out]
        n127 = call <resource>:"Generate Default Project Name and Path.vi"("DNL_MetaDataObj in"=w410) -> ("Project Root"=w419:path, "Project Name"=w418:string, "DNL_MetaDataObj out"=w421:refnum<class "MetaDataObj.lvclass">)  [unwired: 8 in]
        n128 = Unbundle By Name(w393) -> ("AvailableTargets"=w392:refnum<vi>)
        n129 = local write "Project Name"(w418) -> ()
        n130 = local write "Project Root"(w419) -> ()
        n131 = property on="myRIO Device Button" class="myRIO Device Button (strict)"(error in=w380, "Device Code"=u32 0) -> (error out=w379:errorcluster)  [unwired: 1 in, 1 out]
        n132 = property class="RadioBtnsControl (strict)"(reference=w392) -> ("Controls[]"=w391:refnum<vi>[])  [unwired: 1 in, 2 out]
        n133 = To More Specific Class(target class=refnum<class "myRIOMetaDataObj.lvclass"> refnum ("myRIOMetaDataObj.lvclass"), reference=w421) -> (specific class reference=w420:refnum<class "myRIOMetaDataObj.lvclass">)  [unwired: 1 in, 1 out]
        n134 = Index Array(array=w391, index=1) -> (element=w388:refnum<vi>)
        n135 = call "Mapping Channel and Image.vi"("Operation"=T10."Initial") -> ("Channel Info Index Out"=w395:u16)  [unwired: 9 in, 1 out]
        n136 = call <resource>:"CreateDefaultOverlay.vi"("File Prefix"=w417) -> ("Overlay Icon"=w411:refnum<class "Icon.lvclass">)  [unwired: 8 in, 2 out]
        n137 = To More Specific Class(target class=w389, reference=w388) -> (specific class reference=w387:refnum<vi>)  [unwired: 1 in, 1 out]
        n138 = property class="myRIOMetaDataObj.lvclass"(reference=w420, error in=w379, "File Prefix"=w417, "Overlay Icon"=w411) -> (reference out=w403:refnum<class "myRIOMetaDataObj.lvclass">, error out=w402:errorcluster, "Hide Prefix?"=w412:bool, "Hide Icon Overlay?"=w413:bool)
        n139 = Not(x=w412) -> (.not. x?=w416:bool)
        n140 = Not(x=w413) -> (.not. x?=w415:bool)
        n141 = call "SpecificProjectType.vi"("error in (no error)"=w402, "Action"=enum16{"Clear", "Get", "Set"}."Set", "MetaDataObj in"=w403) -> ("error out"=w381:errorcluster, "MetaDataObj out"=w386:refnum<class "MetaDataObj.lvclass">)  [unwired: 5 in, 2 out]
        n142 = call "Get Device Model From Class Path.vi"("MetaDataObj in"=w386) -> ("Dev Ethernet Port"=w384:string, "MetaDataObj Out"=w383:refnum<class "MetaDataObj.lvclass">)  [unwired: 8 in, 1 out]
        n143 = control-ref of="This VI"() -> (w414:refnum<vi>)
        n144 = property on="File Name Prefix (Optional)" class="Str"("Visible"=w416) -> ()  [unwired: 2 in, 2 out]
        n145 = Format Into String(format string="Connected over %s", w384) -> (resulting string=w382:string)  [unwired: 2 in, 1 out]
        n146 = call <resource>:"Show or Hide Spec Page Decorations.vi"("Icon Visible"=w415, "Prefix Visible"=w416, "Spec Page refnum"=w414) -> ()  [unwired: 9 in]
        n147 = property class="Bool"(reference=w387, error in=w381, "BoolText.Text"=w382) -> (reference out=w374:refnum<vi>, error out=w373:errorcluster)
        n148 = Index Array(array=w377, index=0) -> (element=w375:u32)
        n149 = case shown="7885" w375 {
          tunnel: w374 -> [w430 w434]
          tunnel: w373 -> [w429 w433]
          tunnel: [w428 w432] -> w372
          frame Default {
            n150 = property class="Bool"(reference=w430, error in=w429, "DisabledEnum"=T11."Enabled" ("Disabled")) -> (error out=w428:errorcluster)  [unwired: 1 out]
          }
          frame 30853 {
            # "Disable this choice for EL-RIO-CM"
            n151 = property class="Bool"(reference=w434, error in=w433, "DisabledEnum"=T11."Disabled and Grayed Out" ("Disabled")) -> (error out=w432:errorcluster)  [unwired: 1 out]
          }
        }
        n152 = call "SpecificTargetIP.vi"("error in (no error)"=w372, "Action"=enum16{"Clear", "Get", "Set"}."Get") -> ("error out"=w406:errorcluster, "IP or Hostname out"=w407:string)  [unwired: 8 in]
        n153 = Empty String/Path?(string/path=w407) -> (empty?=w408:bool)
        n154 = case shown="False" w408 {
          tunnel: [w436 w457] -> w404
          tunnel: w407 -> [w451 _]
          tunnel: w406 -> [w448 _]
          tunnel: w400 -> [_ _]
          tunnel: w393 -> [w456 w477]
          tunnel: [w446 w467] -> w396
          tunnel: w395 -> [_ _]
          frame False {
            w441 = FALSE ("Visible")
            w446 = AvailableTargets."TargetIP" ("Value (Signaling)")
            w439 = T11."Disabled and Grayed Out" ("Disabled")
            # "The customer had selected a target from myRIO hardware wizard."
            n155 = Unbundle By Name(w456) -> ("AvailableTargets"=w450:refnum<vi>, "Target Tab Control"=w455:refnum<vi>, "IP"=w452:refnum<vi>)
            n156 = property class="RadioBtnsControl (strict)"(reference=w450, error in=w448, "Val(Sgnl)"=w446, "DisabledEnum"=T11."Disabled and Grayed Out" ("Disabled")) -> (error out=w449:errorcluster)  [unwired: 1 out]
            n157 = property class="TabCtl (strict)"(reference=w455, error in=w449, "Value"=enum32{"Target List Page", "IP Config Page"}."IP Config Page") -> (error out=w453:errorcluster)  [unwired: 1 out]
            n158 = property class="Str"(reference=w452, error in=w453, "DisabledEnum"=w439, "Value"=w451) -> (error out=w445:errorcluster)  [unwired: 1 out]
            n159 = property on="FPGA Personality Selector" class="Ring (strict)"(error in=w445, "Val(Sgnl)"=u16 0 ("Value (Signaling)"), "Visible"=w441, "DisabledEnum"=w439) -> (error out=w443:errorcluster)  [unwired: 1 in, 1 out]
            n160 = Not(x=w441) -> (.not. x?=w440:bool)
            n161 = property on="FPGA Personality Indicator" class="Str"(error in=w443, "Value"="" ("FPGA Personality Indicator"), "Visible"=w440, "DisabledEnum"=w439) -> (error out=w438:errorcluster)  [unwired: 1 in, 1 out]
            n162 = property on="FunctionalityArray" class="Arr (strict)"(error in=w438, "Value"=T1[] [] ("FunctionalityArray")) -> (error out=w436:errorcluster)  [unwired: 1 in, 1 out]
          }
          frame True {
            w461 = FALSE
            w460 = T11."Disabled and Grayed Out" ("Disabled")
            w467 = AvailableTargets."USBTarget" ("Value (Signaling)")
            # "The customer try to create the myRIO project from the LV project wizard."
            n163 = Unbundle By Name(w477) -> ("AvailableTargets"=w471:refnum<vi>, "Target Tab Control"=w475:refnum<vi>, "TargetList"=w474:refnum<vi>, "IP"=w476:refnum<vi>)
            n164 = property class="Str"(reference=w476, "Value"="", "DisabledEnum"=T11."Enabled" ("Disabled")) -> (error out=w470:errorcluster)  [unwired: 1 in, 1 out]
            n165 = property class="RadioBtnsControl (strict)"(reference=w471, error in=w470, "Val(Sgnl)"=w467, "DisabledEnum"=T11."Enabled" ("Disabled")) -> (error out=w469:errorcluster)  [unwired: 1 out]
            n166 = property class="TabCtl (strict)"(reference=w475, error in=w469, "Value"=enum32{"Target List Page", "IP Config Page"}."Target List Page" ("Value (Signaling)"), "DisabledEnum"=T11."Enabled" ("Disabled")) -> (error out=w473:errorcluster)  [unwired: 1 out]
            n167 = property class="LstBox (strict)"(reference=w474, error in=w473, "Item Names"=string[] [], "DisabledEnum"=T11."Enabled" ("Disabled"), "Value"=-1) -> (error out=w466:errorcluster)  [unwired: 1 out]
            n168 = Not(x=w461) -> (.not. x?=w459:bool)
            n169 = property on="FPGA Personality Selector" class="Ring (strict)"(error in=w466, "Value"=u16 0 ("Value (Signaling)"), "DisabledEnum"=w460, "Visible"=w461) -> (error out=w463:errorcluster)  [unwired: 1 in, 1 out]
            n170 = property on="FPGA Personality Indicator" class="Str"(error in=w463, "Value"="" ("FPGA Personality Indicator"), "DisabledEnum"=w460, "Visible"=w459) -> (error out=w458:errorcluster)  [unwired: 1 in, 1 out]
            n171 = property on="FunctionalityArray" class="Arr (strict)"(error in=w458, "Value"=T1[] []) -> (error out=w457:errorcluster)  [unwired: 1 in, 1 out]
          }
        }
        n172 = Unbundle By Name(w405) -> ("Show Overlay"=w426:refnum<user-event>, "Update Path"=w425:refnum<user-event>)
        n173 = Generate User Event(user event=w426, event data cluster=w424, error in=w404) -> (error out=w423:errorcluster)  [unwired: 1 in, 1 out]
        n174 = Generate User Event(user event=w425, event data cluster=w424, error in=w423) -> (error out=w397:errorcluster)  [unwired: 1 in, 1 out]
      }
      event "TargetList": Value Change {
        n175 = event-data() -> ()  [unwired: 1 in, 2 out]
        n176 = Unbundle By Name(w497) -> ("AvailableTargets"=w492:refnum<vi>, "TargetList"=w496:refnum<vi>)
        n177 = Unbundle By Name(w500) -> ("ValidateUI"=w499:refnum<user-event>, "UpdateUI"=w484:refnum<user-event>)
        n178 = property class="LstBox (strict)"(reference=w496) -> ("Value"=w495:i32)  [unwired: 1 in, 2 out]
        n179 = property class="RadioBtnsControl (strict)"(reference=w492) -> ("Value"=w489:T3)  [unwired: 1 in, 2 out]
        n180 = case shown="\"NoSpecificTarget\"" w489 {
          tunnel: w493 -> [w504 w508 w511 w516]
          tunnel: [w505 w509 w513 w516] -> w490
          tunnel: w495 -> [w503 w507 w512 _]
          tunnel: [FALSE TRUE FALSE TRUE] -> w494
          tunnel: [_ _ _ w515] -> w491
          frame "USBTarget", Default {
            n181 = Bundle By Name(cluster=w504, "USBTargetList.Value"=w503) -> (w505:T4)
          }
          frame "NoSpecificTarget" {
            n182 = Bundle By Name(cluster=w508, "GenericTargetList.Value"=w507) -> (w509:T4)
          }
          frame "WifiTarget" {
            n183 = Bundle By Name(cluster=w511, "WiFiTargetList.Value"=w512) -> (w513:T4)
          }
          frame "TargetIP" {
            n184 = Unbundle By Name(w516) -> ("IPTargetList.IP Error Out"=w515:errorcluster)
          }
        }
        n185 = Generate User Event(user event=w499, event data cluster=w491, error in=w498) -> (error out=w486:errorcluster)  [unwired: 1 in, 1 out]
        n186 = Generate User Event(user event=w484, event data cluster=variant ("event data"), error in=w486) -> (error out=w485:errorcluster)  [unwired: 1 in, 1 out]
      }
      event "IP": Value Change {
        n187 = event-data() -> ("NewVal"=w525:string)  [unwired: 1 in]
        n188 = call "ValidateIPorHostname.vi"("IP Address or Hostname"=w525) -> ("error out"=w523:errorcluster, "Valid?"=w524:bool)  [unwired: 9 in]
        n189 = case shown="True" w524 {
          tunnel: w532 -> [_ w546]
          tunnel: [T6[] [] w545] -> w529
          tunnel: [w538 w544] -> w528
          tunnel: w525 -> [_ w543]
          tunnel: w523 -> [w538 _]
          tunnel: w518 -> [_ w540]
          frame False {
          }
          frame True {
            n190 = flat-sequence {
              tunnel: w543 -> [w560]
              tunnel: [w560] -> w556
              tunnel: [w559] -> w555
              tunnel: w546 -> [w558]
              tunnel: w540 -> [w557]
              tunnel: [w557] -> w541
              tunnel: w556 -> [w565]
              tunnel: [w565] -> w554
              tunnel: w555 -> [w564]
              tunnel: [w564] -> w553
              tunnel: [w562] -> w552
              tunnel: [w561] -> w542
              tunnel: w541 -> [w561]
              tunnel: [w571] -> w545
              tunnel: w554 -> [w572]
              tunnel: [w570] -> w551
              tunnel: [w569] -> w550
              tunnel: w553 -> [w569]
              tunnel: w552 -> [w567]
              tunnel: [w567] -> w549
              tunnel: w542 -> [w566]
              tunnel: w551 -> [w574]
              tunnel: w550 -> [w576]
              tunnel: w546 -> [w575]
              tunnel: [w574] -> w548
              tunnel: [w573] -> w547
              tunnel: w549 -> [w573]
              tunnel: [w579] -> w544
              tunnel: w548 -> [w579]
              tunnel: w547 -> [w577]
              frame #0 {
                n191 = call <vilib>:"Set Busy.vi"("VI reference (current VI)"=w558) -> ("error out"=w559:errorcluster)  [unwired: 9 in, 1 out]
              }
              frame #1 {
                n192 = global read "InternalErrorCodes.vi" "ConnectTargetByIP"() -> (w563:string)
                n193 = property on="WarningMsg" class="Str"("Value"=w563) -> (error out=w562:errorcluster)  [unwired: 2 in, 1 out]
              }
              frame #2 {
                n194 = call "CheckRTTargetModel.vi"("Supported Devices"=w566, "IP or Hostname"=w572) -> ("error out"=w570:errorcluster, "RT Target Info"=w568:T6)  [unwired: 8 in]
                n195 = Build Array(w568) -> (w571:T6[])
              }
              frame #3 {
                n196 = call <vilib>:"Unset Busy.vi"("error in (no error)"=w576, "VI reference (current VI)"=w575) -> ()  [unwired: 9 in, 1 out]
              }
              frame #4 {
                n197 = property on="WarningMsg" class="Str"(error in=w577, "Value"="") -> ()  [unwired: 1 in, 2 out]
              }
            }
          }
        }
        n198 = Unbundle By Name(w535) -> ("ValidateUI"=w534:refnum<user-event>, "UpdateUI"=w519:refnum<user-event>)
        n199 = Generate User Event(user event=w534, event data cluster=w528, error in=w533) -> (error out=w521:errorcluster)  [unwired: 1 in, 1 out]
        n200 = Generate User Event(user event=w519, event data cluster=variant ("event data"), error in=w521) -> (error out=w520:errorcluster)  [unwired: 1 in, 1 out]
        n201 = Bundle By Name(cluster=w530, "IPTargetList.IP Error Out"=w528, "IPTargetList.Target RT Info List"=w529) -> (w527:T4)
      }
      event "File Name Prefix (Optional)": Value Change {
        w584 = FALSE ("event data")
        n202 = event-data() -> ("NewVal"=w593:string)  [unwired: 1 in]
        n203 = Unbundle By Name(w588) -> ("Update Path"=w586:refnum<user-event>, "Show Overlay"=w585:refnum<user-event>)
        n204 = Generate User Event "\"Update Path\" event"(user event=w586, event data cluster=w584, error in=w583) -> (error out=w587:errorcluster)  [unwired: 1 in, 1 out]
        n205 = Generate User Event "\"Show Overlay\" event"(user event=w585, event data cluster=w584, error in=w587) -> (error out=w582:errorcluster)  [unwired: 1 in, 1 out]
        n206 = case shown="False" w590 {
          tunnel: w593 -> [w597 _]
          tunnel: w592 -> [w596 w598]
          tunnel: [w595 w598] -> w591
          frame False {
            n207 = call <resource>:"CreateDefaultOverlay.vi"("File Prefix"=w597) -> ("Overlay Icon"=w594:refnum<class "Icon.lvclass">)  [unwired: 8 in, 2 out]
            n208 = property class="MetaDataObj.lvclass"(reference=w596, "Overlay Icon"=w594) -> (reference out=w595:refnum<class "MetaDataObj.lvclass">)  [unwired: 1 in, 1 out]
          }
          frame True {
          }
        }
      }
      event User Event {
        n209 = event-data() -> ()  [unwired: 1 in, 1 out]
        n210 = property on="AvailableTargets" class="RadioBtnsControl (strict)"() -> ("Value"=w599:T3)  [unwired: 2 in, 2 out]
        n211 = call "UpdatePath.vi"("File Name Prefix (Optional)"="File Name Prefix (Optional)", "Project Root"="Project Root", "Project Name"="Project Name", "MetaDataObj in"=w603) -> ("error out"=w601:errorcluster, "MetaDataObj out"=w602:refnum<class "MetaDataObj.lvclass">)  [unwired: 6 in]
        n212 = Unbundle By Name(w612) -> ("ValidateUI"=w611:refnum<user-event>)
        n213 = case shown="\"TargetIP\"" w599 {
          tunnel: w607 -> [_ w619]
          tunnel: w601 -> [w615 w617]
          tunnel: [w615 w616] -> w600
          frame Default {
          }
          frame "TargetIP" {
            n214 = Unbundle By Name(w619) -> ("IPTargetList.IP Error Out"=w618:errorcluster)
            n215 = Merge Errors(w618, w617) -> (w616:errorcluster)
          }
        }
        n216 = Generate User Event(user event=w611, event data cluster=w600, error in=w610) -> (error out=w609:errorcluster)  [unwired: 1 in, 1 out]
      }
      event Key Down? {
        n217 = event-data() -> ("Char"=w642:i16, "PlatMods.Shift"=w641:bool)  [unwired: 1 in, 1 out]
        n218 = Unbundle By Name(w634) -> ("\"Tab Forward To\" Refnum"=w640:refnum<vi>, "\"Tab Backward To\" Refnum"=w639:refnum<vi>)
        n219 = Unbundle By Name(w633) -> ("Project Name"=w627:refnum<vi>, "AvailableTargets"=w625:refnum<vi>, "Refresh"=w623:refnum<vi>, "TargetList"=w622:refnum<vi>, "IP"=w621:refnum<vi>)
        n220 = property class="RadioBtnsControl (strict)"(reference=w625) -> ("Value"=w624:T3)  [unwired: 1 in, 2 out]
        n221 = case shown="\"TargetIP\"" w624 {
          tunnel: w623 -> [w644 _ _]
          tunnel: w622 -> [_ w645 _]
          tunnel: w621 -> [_ _ w646]
          tunnel: [w644 w645 w646] -> w620
          frame "USBTarget", "WifiTarget", Default {
          }
          frame "NoSpecificTarget" {
          }
          frame "TargetIP" {
          }
        }
        n222 = control-ref of="FPGA Personality Selector"() -> (w626:refnum<vi>)
        n223 = property class="Ring (strict)"(reference=w626) -> (reference out=w629:refnum<vi>, "DisabledEnum"=w630:T11)  [unwired: 1 in, 1 out]
        n224 = case shown="\"Disabled\", Default" w630 {
          tunnel: w629 -> [w647 _]
          tunnel: [w647 w648] -> w628
          tunnel: w620 -> [_ w648]
          frame "Enabled" {
          }
          frame "Disabled", Default {
          }
        }
        n225 = call <resource>:"HandleInnerVITabbing.vi"("Tab Backward To"=w639, "Tab Forward To"=w640, "Char"=w642, "Last Control"=w628, "First Control"=w627, "Shift"=w641) -> ("Discard"=w643:bool)  [unwired: 5 in]
        n226 = event-data("Discard?"=w643) -> ()  [unwired: 1 in, 1 out]
      }
      event "Refresh Button": Value Change {
        n227 = event-data() -> ()  [unwired: 1 in, 1 out]
        n228 = Unbundle By Name(w658) -> ("ValidateUI"=w657:refnum<user-event>)
        n229 = call "Refresh Target List.vi"("Supported Devices"=w649, "OwningVI Ref"=w654, "UI Ref Cluster"=w655, "Target Info Cache"=w652) -> ("error out"=w653:errorcluster, "Target Info Cache Output"=w651:T4)  [unwired: 6 in]
        n230 = Generate User Event(user event=w657, event data cluster=w653, error in=w660) -> (error out=w659:errorcluster)  [unwired: 1 in, 1 out]
      }
      event "IP": Key Down {
        n231 = event-data() -> ()  [unwired: 1 in, 5 out]
      }
      event "FPGA Personality Selector": Value Change {
        w678 = 12 ("y")
        n232 = event-data() -> ("CtlRef"=w691:refnum<vi>, "NewVal"=w689:u16)  [unwired: 1 in]
        n233 = property on="Property Node" class="Ring (strict)"(reference=w691) -> ("Strings []"=w690:string[])  [unwired: 1 in, 2 out]
        n234 = Index Array(array=w690, index=w689) -> (element=w688:string)
        n235 = call "GetImageIndex.vi"("Supported Devices"=w669, "TargetInfoHistory"=w686, "AvailableTarget"=w687) -> ("ProdID"=w685:u32)  [unwired: 8 in]
        n236 = call "GetFPGAPersonalityDescription.vi"("FPGA Personality Name"=w688, "ProdID"=w685) -> ("error out"=w683:errorcluster, "Help Link"=w681:string, "CHM Link"=w680:string, "Description"=w674:string, "IO Info"=w682:T13[])  [unwired: 5 in]
        n237 = case shown="No Error" w683 {
          tunnel: w682 -> [w717 _]
          tunnel: [w719 _] -> w684
          tunnel: [w716 0] -> w677
          tunnel: w681 -> [w714 _]
          tunnel: w680 -> [w715 _]
          tunnel: w674 -> [w700 _]
          frame No Error {
            n238 = Array Size(array=w717) -> (size(s)=w716:i32)
            n239 = for {
              tunnel: w717 -> [w733] mode=indexing
              shift-right: [w730] -> w719
              shift-left: T1[] [] -> [w731]
              n240 = Unbundle By Name(w733) -> ("Channel Info Index"=w724:i8, "IO Number"=w732:i8)
              n241 = Number To Decimal String(number=w732) -> (decimal integer string=w726:string)  [unwired: 1 in]
              n242 = call "Mapping Channel and Image.vi"("Channel Info Index In"=w724, "Operation"=T10."Get Channel Info by Index") -> ("Channel Info"=w723:T14)  [unwired: 8 in, 1 out]
              n243 = Unbundle By Name(w723) -> ("Channel Shortcut"=w721:string, "Channl Image Index"=w722:u16)
              n244 = Concatenate Strings(w726, "\r", w721) -> (w727:string)
              n245 = Bundle By Name(cluster=T1 {"myRIOMode Functionality"=0, "SupportNumber"=""} ("Cluster"), "myRIOMode Functionality"=w722, "SupportNumber"=w727) -> (w729:T1)
              n246 = Build Array (concatenate)(w731, w729) -> (w730:T1[])
            }
            n247 = Concatenate Strings(w715, "/", w714) -> (w698:string)
            n248 = control-ref of="Mode Help Link"() -> (w699:refnum<vi>)
            n249 = String Length(string=w700) -> (length=w706:i32)
            n250 = call <vilib>:"Space Constant.vi"() -> ("String"=w702:string)
            n251 = Increment(x=w706) -> (x+1=w701:i32)
            n252 = Concatenate Strings(w700, w702, "Learn more") -> (w710:string)
            n253 = Add(x=w701, y=10) -> (x+y=w705:i32)
            n254 = property class="Str"(reference=w699, "Value"=w710, "Text.Selection Start"=u32 0 ("Text.Selection:Start"), "Text.Selection End"=w701, "Text.FontUnder"=FALSE ("Text.Font:Underline"), "Text.FontColor"=u32 0 ("Text.Text Colors:Text Color"), "Text.Selection Start"=w701, "Text.Selection End"=w705, "Text.FontUnder"=TRUE ("Text.Font:Underline"), "Text.FontColor"=u32 8191 ("Text.Text Colors:Text Color"), "Desc"=w698) -> ()  [unwired: 1 in, 2 out]
          }
          frame Error {
          }
        }
        n255 = Greater?(x=w677, y=w678) -> (0:w679:bool)
        n256 = property on="FunctionalityArray" class="Arr (strict)"("Visible"=FALSE) -> (error out=w673:errorcluster)  [unwired: 2 in, 1 out]
        n257 = case shown="False" w679 {
          tunnel: w678 -> [_ w697]
          tunnel: [w696 w697] -> w676
          tunnel: w677 -> [w696 _]
          frame False {
          }
          frame True {
          }
        }
        n258 = property on="FunctionalityArray" class="Arr (strict)"(error in=w673, "Value"=w684, "Number of Columns"=w676, "HorizScroll"=w679, "DisabledEnum"=T11."Enabled" ("Disabled")) -> (error out=w672:errorcluster)  [unwired: 1 in, 1 out]
        n259 = property on="FunctionalityArray" class="Arr (strict)"(error in=w672, "Visible"=TRUE) -> ()  [unwired: 1 in, 2 out]
      }
      event User Event {
        n260 = event-data() -> ()  [unwired: 1 in, 1 out]
        n261 = call "GetImageIndex.vi"("Supported Devices"=w751, "TargetInfoHistory"=w759, "AvailableTarget"=w758) -> ("ProdID"=w738:u32)  [unwired: 8 in]
        n262 = Equal To 0?(x=w738) -> (x = 0?=w750:bool)
        n263 = call <vilib>:"Get Target Name by PID.vi"("Full Name?"=TRUE, "Device Model"=w738) -> ("Device Model Str"=w739:string)  [unwired: 8 in, 1 out]
        n264 = property on="myRIO Device Button" class="myRIO Device Button (strict)"("Device Code"=w738, "TipStrip"=w739) -> ()  [unwired: 2 in, 2 out]
        n265 = case shown="False" w750 {
          tunnel: [w772 w787] -> w735
          tunnel: w757 -> [w786 _]
          tunnel: [w763 u16 0 ("Value")] -> w754
          tunnel: [w769 w789] -> w753
          tunnel: ["" ("Mode Help Link") "" ("Mode Help Link")] -> w752
          tunnel: w738 -> [w783 _]
          tunnel: [w773 FALSE] -> w745
          tunnel: [w776 w790] -> w747
          tunnel: [w771 w787] -> w736
          frame False {
            w770 = "Default" ("f")
            w771 = T11."Enabled" ("Disabled")
            n266 = property class="MetaDataObj.lvclass"(reference=w786) -> (reference out=w781:refnum<class "MetaDataObj.lvclass">, "Title"=w782:string)  [unwired: 1 in, 1 out]
            n267 = call "GetFPGAPersonalityListInfo.vi"("MetaDataObj in"=w781, "Project Title"=w782, "ProdID"=w783) -> ("Available FPGA Tags"=w785:string[], "Available FPGA Personalities"=w768:string[], "Index for Default Personality"=w765:u16)  [unwired: 4 in, 2 out]
            n268 = property on="Personality Tags" class="Ring (strict)"("Strings []"=w785) -> ()  [unwired: 2 in, 2 out]
            n269 = Array Size(array=w768) -> (size(s)=w778:i32)
            n270 = Greater?(x=w778, y=1) -> (0:w773:bool)
            n271 = Not Equal To 0?(x=w778) -> (x != 0?=w766:bool)
            n272 = Select(t=w765, s=w773, f=u16 0) -> (s? t:f=w779:u16)
            n273 = Select(t=w765, s=w766, f=u16 0) -> (s? t:f=w763:u16)
            n274 = Index Array(array=w768, index=w779) -> (element=w775:string)
            n275 = Build Array(w770) -> (w767:string[])
            n276 = Select(t=w768, s=w766, f=w767) -> (s? t:f=w769:string[])
            n277 = Select(t=w775, s=w766, f=w770) -> (s? t:f=w776:string)
            n278 = Select(t=w771, s=w773, f=T11."Disabled" ("Disabled")) -> (s? t:f=w772:T11)
          }
          frame True {
            w789 = string[] ["Select a Target ... "] ("Strings []")
            w787 = T11."Disabled and Grayed Out" ("Disabled")
            n279 = Index Array(array=w789, index=0) -> (element=w790:string)
          }
        }
        n280 = property on="Mode Help Link" class="Str"("DisabledEnum"=w736, "Value"=w752) -> ()  [unwired: 2 in, 2 out]
        n281 = property on="FPGA Personality Selector" class="Ring (strict)"("DisabledEnum"=w735, "Val(Sgnl)"=w754, "Strings []"=w753, "Visible"=w745) -> (error out=w749:errorcluster)  [unwired: 2 in, 1 out]
        n282 = Subtract(x=T11."Disabled" ("y"), y=w735) -> (x-y=w740:u8)
        n283 = Equal?(x=w735, y=T11."Disabled and Grayed Out") -> (x = y?=w744:bool)
        n284 = Not(x=w745) -> (.not. x?=w746:bool)
        n285 = Select(t=w735, s=w744, f=w740) -> (s? t:f=w743:u8)
        n286 = property on="FPGA Personality Indicator" class="Str"(error in=w749, "Value"=w747, "Visible"=w746, "DisabledEnum"=w743) -> (error out=w748:errorcluster)  [unwired: 1 in, 1 out]
        n287 = property on="FunctionalityArray" class="Arr (strict)"(error in=w748, "Number of Columns"=u32 0, "Value"=T1[] [] ("FunctionalityArray")) -> ()  [unwired: 1 in, 2 out]
      }
      event "Project Name", "Project Root", "File Name Prefix (Optional)", "Target Tab Control", "Refresh Button", "IP", "TargetList", "WarningMsg", "FunctionalityArray", "Personality Tags", "myRIO Device Button", "FPGA Personality Indicator": Mouse Down? {
        # "Disable right click event and middle button click event of mouse"
        n288 = event-data() -> ("Button"=w799:u16)  [unwired: 1 in, 7 out]
        n289 = Equal?(x=u16 2, y=w799) -> (x = y?=w796:bool)
        n290 = Equal?(x=w799, y=u16 3) -> (x = y?=w795:bool)
        n291 = Or(x=w796, y=w795) -> (x .or. y?=w794:bool)
        n292 = event-data("Discard?"=w794) -> ()  [unwired: 1 in, 1 out]
      }
      event "Mode Help Link": Mouse Down {
        # "The chm and html should be defined by the FPGA personality definition file (*.xml) in the folder \"vi.lib\\myRIO\\FPGA\\bitfiles\"."
        n293 = event-data() -> ()  [unwired: 1 in, 8 out]
        n294 = property on="Mode Help Link" class="Str"() -> ("DisabledEnum"=w807:T11, "Desc"=w806:string)  [unwired: 2 in, 2 out]
        n295 = case shown="\"Enabled\"" w807 {
          tunnel: w806 -> [w817 _]
          frame "Enabled" {
            n296 = Search/Split String(string=w817, search string/char (-)="/") -> (substring before match=w814:string, match + rest of string=w819:string)  [unwired: 1 in, 1 out]
            n297 = String Subset(string=w819, offset (0)=1) -> (substring=w816:string)  [unwired: 1 in]
            n298 = Empty String/Path?(string/path=w814) -> (empty?=w815:bool)
            n299 = case shown="True" w815 {
              tunnel: w814 -> [w822 _]
              tunnel: w816 -> [w821 w823]
              frame False {
                # "Open CHM"
                n300 = call <helpdir>:"_LaunchHelp.vi"("CHM or HLP filename (lvdialog.chm)"=w822, "HTML filename"=w821) -> ()  [unwired: 1 in, 5 out]
              }
              frame True {
                # "Open URL"
                n301 = call-poly <vilib>:"Open URL in Default Browser.vi"("URL"=w823) -> ()  [unwired: 5 in, 2 out]
              }
            }
          }
          frame "Disabled", Default {
          }
        }
      }
      event "FunctionalityArray": Mouse Move {
        n302 = event-data() -> ("Coords"=w831:T15)  [unwired: 1 in, 4 out]
        n303 = control-ref of="FunctionalityArray"() -> (w824:refnum<vi>)
        n304 = control-ref of="FPGA Personality Selector"() -> (w830:refnum<vi>)
        n305 = control-ref of="FPGA Personality Indicator"() -> (w828:refnum<vi>)
        n306 = Unbundle By Name(w831) -> ("Horizontal"=w829:i32)
        n307 = property class="Ring (strict)"(reference=w830) -> ("DisabledEnum"=w827:T11)  [unwired: 1 in, 2 out]
        n308 = property class="Str"(reference=w828) -> ("DisabledEnum"=w826:T11)  [unwired: 1 in, 2 out]
        n309 = And(x=w827, y=w826) -> (x .and. y?=w825:i32)
        n310 = case shown="Default" w825 {
          tunnel: w829 -> [w858 _]
          tunnel: w824 -> [w838 w865]
          frame 0 {
            # "If the mouse is in the middle part of the icon, show tthe tool tip, otherwise, clean up the tooltip"
            n311 = property class="Arr (strict)"(reference=w838) -> (reference out=w857:refnum<vi>, "Left"=w856:i32, "Array Element.Width"=w854:u32, "Value"=w862:T1[], "Index Values"=w844:u32[])  [unwired: 1 in, 1 out]
            n312 = Subtract(x=w858, y=w856) -> (x-y=w845:i32)
            n313 = Index Array(array=w844, index=0) -> (element=w840:u32)
            n314 = Quotient & Remainder(x=w845, y=w854) -> (x-y*floor(x/y)=w855:u32, floor(x/y)=w841:u32)
            n315 = Add(x=w840, y=w841) -> (x+y=w842:u32)
            n316 = Index Array(array=w862, index=w842) -> (element=w861:T1)
            n317 = Divide(x=w855, y=w854) -> (x/y=w852:dbl)
            n318 = Unbundle By Name(w861) -> ("myRIOMode Functionality"=w860:u16)
            n319 = Greater Or Equal?(x=w852, y=0.15) -> (x >= y?=w850:bool)
            n320 = Less Or Equal?(x=w852, y=0.85) -> (x <= y?=w849:bool)
            n321 = And(x=w850, y=w849) -> (x .and. y?=w848:bool)
            n322 = call "Mapping Channel and Image.vi"("Channel Info Index In"=w860, "Operation"=T10."Get Channel Info by Img Index") -> ("Channel Info"=w859:T14)  [unwired: 8 in, 1 out]
            n323 = Unbundle By Name(w859) -> ("Channel Description"=w839:string)
            n324 = case shown="False" w848 {
              tunnel: w839 -> [_ w864]
              tunnel: ["" ("Channel Description") w864] -> w847
              frame False {
              }
              frame True {
              }
            }
            n325 = property class="Arr (strict)"(reference=w857, "TipStrip"=w847) -> ()  [unwired: 1 in, 2 out]
          }
          frame Default {
            n326 = property class="Arr (strict)"(reference=w865, "TipStrip"="" ("Tip Strip")) -> ()  [unwired: 1 in, 2 out]
          }
        }
      }
      event "Mode Help Link": Mouse Enter; "Mode Help Link": Mouse Leave {
        n327 = event-data() -> ("Type"=w869:T16)  [unwired: 1 in, 1 out]
        n328 = case shown="\"Mouse Leave\", Default" w869 {
          tunnel: [u16 0 ("icon") u16 6 ("icon")] -> w867
          frame "Mouse Leave", Default {
          }
          frame "Mouse Enter" {
          }
        }
        n329 = call-poly <vilib>:"Set Cursor.vi"("VI reference (current VI)"=w868, "icon"=w867) -> ()  [unwired: 8 in, 2 out]
      }
    }
    n330 = Or(x=w65, y=w56) -> (x .or. y?=w71:bool)
  }
  "MetaDataObj out" <- w51
  n331 = Unbundle By Name(w31) -> ("InitUI"=w28:refnum<user-event>, "ValidateUI"=w27:refnum<user-event>, "Show Overlay"=w26:refnum<user-event>, "Update Path"=w25:refnum<user-event>, "UpdateUI"=w1:refnum<user-event>)
  n332 = Unregister For Events(event registration refnum=w18, error in=w47) -> (error out=w52:errorcluster)
  n333 = Destroy User Event(user event=w28, error in=w52) -> (error out=w50:errorcluster)
  n334 = Destroy User Event(user event=w27, error in=w50) -> (error out=w30:errorcluster)
  n335 = Destroy User Event(user event=w26, error in=w30) -> (error out=w29:errorcluster)
  n336 = Destroy User Event(user event=w25, error in=w29) -> (error out=w2:errorcluster)
  n337 = Destroy User Event(user event=w1, error in=w2) -> ()  [unwired: 1 out]
